vi "--Autonomous Independent.vi"() -> ()   [LabVIEW 2012]
doc: "This VI is called when autonomous begins, and will automatically be terminated when autonomous ends. You can carry out timed or sensor driven robot movement independently without needing to return to the caller."
uses:
  <vilib>/Rock Robotics/WPI/Relay/WPI_RelayValue.ctl
  <vilib>/Rock Robotics/WPI/Solenoid/WPI_SolenoidValue.ctl
  Robot Global Data.vi
  <vilib>/Rock Robotics/WPI/RobotDrive/WPI_RobotDriveGetSetRefNum.vi
  <vilib>/Rock Robotics/WPI/Solenoid/WPI_SolenoidSetEnum.vi
  <vilib>/Rock Robotics/WPI/Joystick/WPI_JoystickGetSetRefNum.vi
  <vilib>/addons/control/pid/NI_PID_pid.lvlib
  <vilib>/addons/control/pid/pid.llb/PID (DBL).vi
panel:
  in  "Auton Launch Reduction":dbl
  in  "Quicklaunch State":T1(ring)
  in  "Fast-Slow Variable":dbl
  out "Launch Wait tick":dbl
  out "Time Between tick":dbl
  in  "Time Between Launches":dbl=2000.0
  in  "Charge Up Time":dbl=4000.0
  out "Charge Up tick":dbl
  in  "Launch Wait Time":dbl=500.0
  in  "Turn wait time fr":dbl=250.0
  in  "Drive wait time fr":dbl=400.0
  in  "Turn wait time fl":dbl=250.0
  in  "Drive wait time fl":dbl=400.0
  in  "Drive wait time cl":dbl=400.0
  in  "Turn wait time cr":dbl=250.0
  in  "Drive wait time cr":dbl=400.0
  in  "Time between launches":dbl=1000.0
  in  "Launcher Charge time":dbl=5000.0
  in  "Drive PID gains":T2={"proportional gain (Kc)"=1.0, "integral time (Ti, min)"=0.01, "derivative time (Td, min)"=0.0} {"derivative time (Td, min)" format="%.3f"; "integral time (Ti, min)" format="%.3f"; "proportional gain (Kc)" format="%.3f"}
  in  "Turn wait time cl":dbl=250.0
  out "Field Position":enum16{"Corner", "Middle"}(ring)
  in  "Turn PID gains":T2={"proportional gain (Kc)"=1.0, "integral time (Ti, min)"=0.01, "derivative time (Td, min)"=0.0} {"derivative time (Td, min)" format="%.3f"; "integral time (Ti, min)" format="%.3f"; "proportional gain (Kc)" format="%.3f"}
  in  "Sweet Spot":dbl
  out "tick":dbl
  in  "-Fast-Slow Variable":dbl=2.0
  out "Numeric 0":dbl
  out "Current Movement, for debugging":T3 {"Y Joystick Value" scale=1.0..-1.0; "X Joystick Value" scale=-1.0..1.0}
  in  "Array of robot movements":T4(array[cluster]) {"Y Joystick Value" scale=1.0..-1.0; "X Joystick Value" scale=-1.0..1.0}
  # "Be sure to right-click and choose Data Operations>>Make Current Value default if you want to save the array values with the VI"
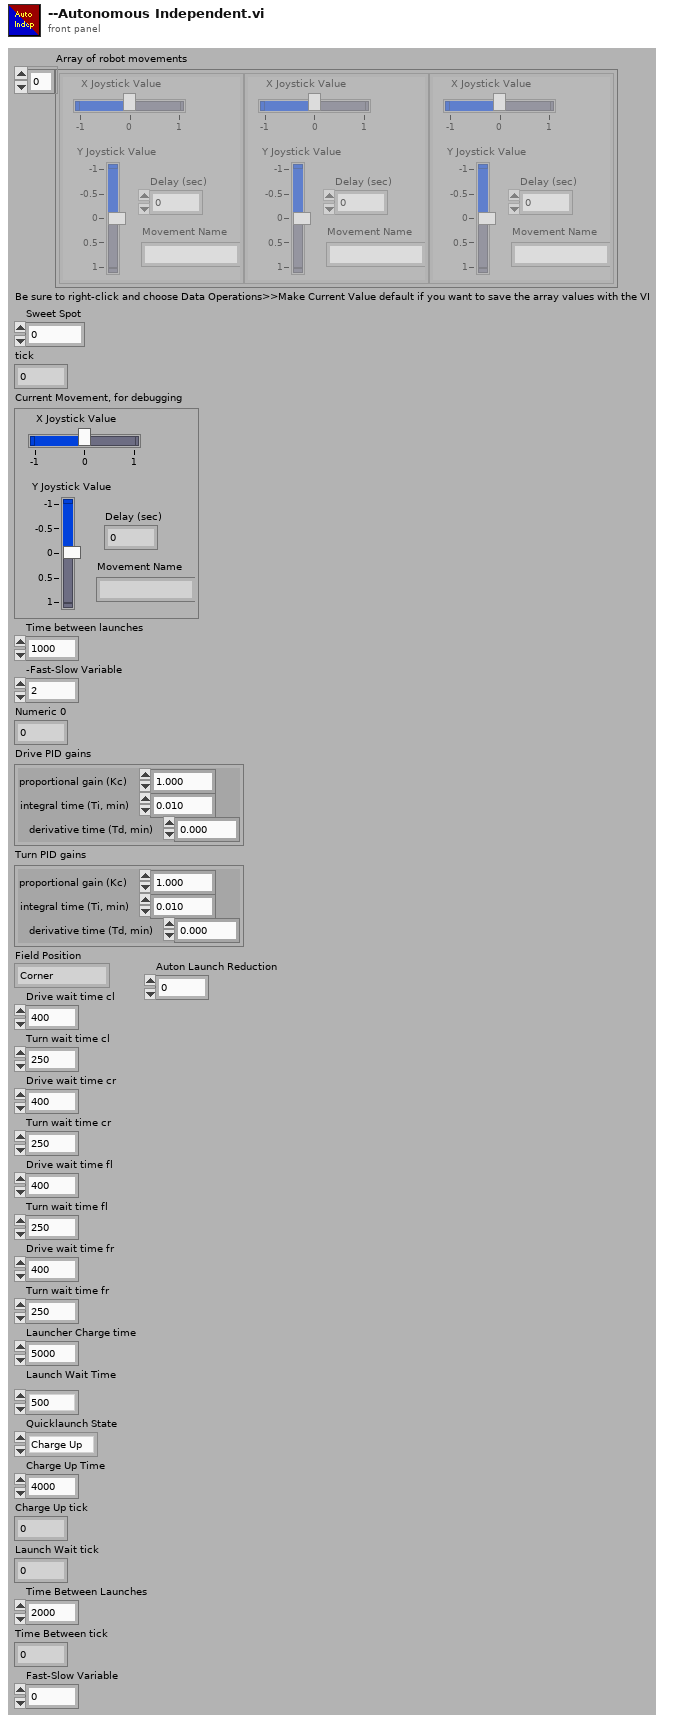
[diagram p1: front panel]
types:
  T1 = enum16{"Charge Up ", "Fire 1", "wait1", "Fire 2", "wait2", "Fire 3", "wait3", "Fire 4"}
  T2 = cluster{"proportional gain (Kc)":dbl, "integral time (Ti, min)":dbl, "derivative time (Td, min)":dbl}
  T3 = cluster{"X Joystick Value":dbl, "Y Joystick Value":dbl, "Delay (sec)":dbl, "Movement Name":string}
  T4 = cluster{"X Joystick Value":dbl, "Y Joystick Value":dbl, "Delay (sec)":dbl, "Movement Name":string}[]
  T5 = typedef "WPI_JoystickDevRef.ctl" = cluster{"Device":T6}
  T6 = typedef "WPI_JoystickDeviceEnum.ctl" = enum16{"USB 1", "USB 2", "USB 3", "USB 4", "Kinect 1", "Kinect 2"}
  T7 = cluster{"axis 1 (x)":dbl, "axis 2 (y)":dbl, "axis 3 (throttle)":dbl, "axis 4":dbl, "axis 5":dbl, "axis 6":dbl}
  T8 = typedef "WPI_SolenoidValue.ctl" = enum16{"Off", "On", "Forward", "Reverse"}
  T9 = typedef "WPI_RobotDriveDevRef.ctl" = cluster{"DevStatus":errorcluster, "Motors[]":T10[], "Square Inputs":bool, "Max Output":dbl, "Isochronous":bool}
  T10 = typedef "WPI_MotorControlDeviceRef.ctl" = cluster{"DeviceStatus":errorcluster, "Type":enum16{"PWM", "CAN"}, "PWM":cluster{"Digital Module":T11, "PWM Channel":T12, "DeadBand":T13}, "CAN":cluster{"Device Number":u8, "Control Mode":T14, "Semaphore":T15, "Max Vout":dbl}, "Invert":bool, "TransformRef":T16, "InvTransformRef":T16}
  T11 = typedef "FPGA_TypedefDigitalModule.ctl" = enum16{"Digital Module 1", "Digital Module 2"}
  T12 = typedef "FPGA_DIOPWMChannel.ctl" = enum8{"PWM 1", "PWM 2", "PWM 3", "PWM 4", "PWM 5", "PWM 6", "PWM 7", "PWM 8", "PWM 9", "PWM 10", "Invalid"}
  T13 = typedef "WPI_PWMDeadband.ctl" = cluster{"Name":string, "maxPositivePwm":i32, "minPositivePwm":i32, "centerPwm":i32, "maxNegativePwm":i32, "minNegativePwm":i32, "angularRange":u16}
  T14 = typedef "WPI_CANJaguar_ControlMode.ctl" = enum8{"Percent VBus", "Current", "Speed", "Position", "Voltage"}
  T15 = typedef "Semaphore RefNum" = refnum<k1>
  T16 = typedef "WPI_PWMTransform_ConPane.ctl" = refnum<vi>
  T17 = cluster{"Center Position":cluster{"X":dbl, "Y":dbl}, "Distance (ft)":dbl, "Center":bool}[]
  T18 = cluster{"Target Info[0]":cluster{"Center Position":cluster{"X":dbl, "Y":dbl}, "Distance (ft)":dbl, "Center":bool}, "Target Info[1]":cluster{"Center Position":cluster{"X":dbl, "Y":dbl}, "Distance (ft)":dbl, "Center":bool}, "Target Info[2]":cluster{"Center Position":cluster{"X":dbl, "Y":dbl}, "Distance (ft)":dbl, "Center":bool}, "Target Info[3]":cluster{"Center Position":cluster{"X":dbl, "Y":dbl}, "Distance (ft)":dbl, "Center":bool}, "Target Info[4]":cluster{"Center Position":cluster{"X":dbl, "Y":dbl}, "Distance (ft)":dbl, "Center":bool}, "Target Info[5]":cluster{"Center Position":cluster{"X":dbl, "Y":dbl}, "Distance (ft)":dbl, "Center":bool}, "Target Info[6]":cluster{"Center Position":cluster{"X":dbl, "Y":dbl}, "Distance (ft)":dbl, "Center":bool}, "Target Info[7]":cluster{"Center Position":cluster{"X":dbl, "Y":dbl}, "Distance (ft)":dbl, "Center":bool}, "Target Info[8]":cluster{"Center Position":cluster{"X":dbl, "Y":dbl}, "Distance (ft)":dbl, "Center":bool}}
  T19 = cluster{"Center Position":cluster{"X":dbl, "Y":dbl}, "Distance (ft)":dbl, "Center":bool}
  T20 = typedef "WPI_SolenoidDevRef.ctl" = cluster{"DevStatus":errorcluster, "Solenoid Module":T21, "Forward Solenoid Channel":T22, "Reverse Solenoid Channel":T22}
  T21 = typedef "FPGA_TypedefSolenoidModule.ctl" = enum16{"Solenoid Module 1", "Solenoid Module 2"}
  T22 = typedef "WPI_SolenoidChannel.ctl" = enum8{"Solenoid 1", "Solenoid 2", "Solenoid 3", "Solenoid 4", "Solenoid 5", "Solenoid 6", "Solenoid 7", "Solenoid 8", "Invalid"}
  T23 = typedef "WPI_RelayValue.ctl" = enum16{"Off", "On", "Forward", "Reverse"}
  T24 = typedef "WPI_RelayDevRef.ctl" = cluster{"DevStatus":errorcluster, "Relay Channel":T25, "Digital Module":T11, "Relay Direction":T26}
  T25 = typedef "FPGA_DIORelayChannel.ctl" = enum8{"Relay 1", "Relay 2", "Relay 3", "Relay 4", "Relay 5", "Relay 6", "Relay 7", "Relay 8", "Invalid"}
  T26 = typedef "WPI_RelayDirection.ctl" = enum16{"Both directions", "Forward only", "Reverse only"}
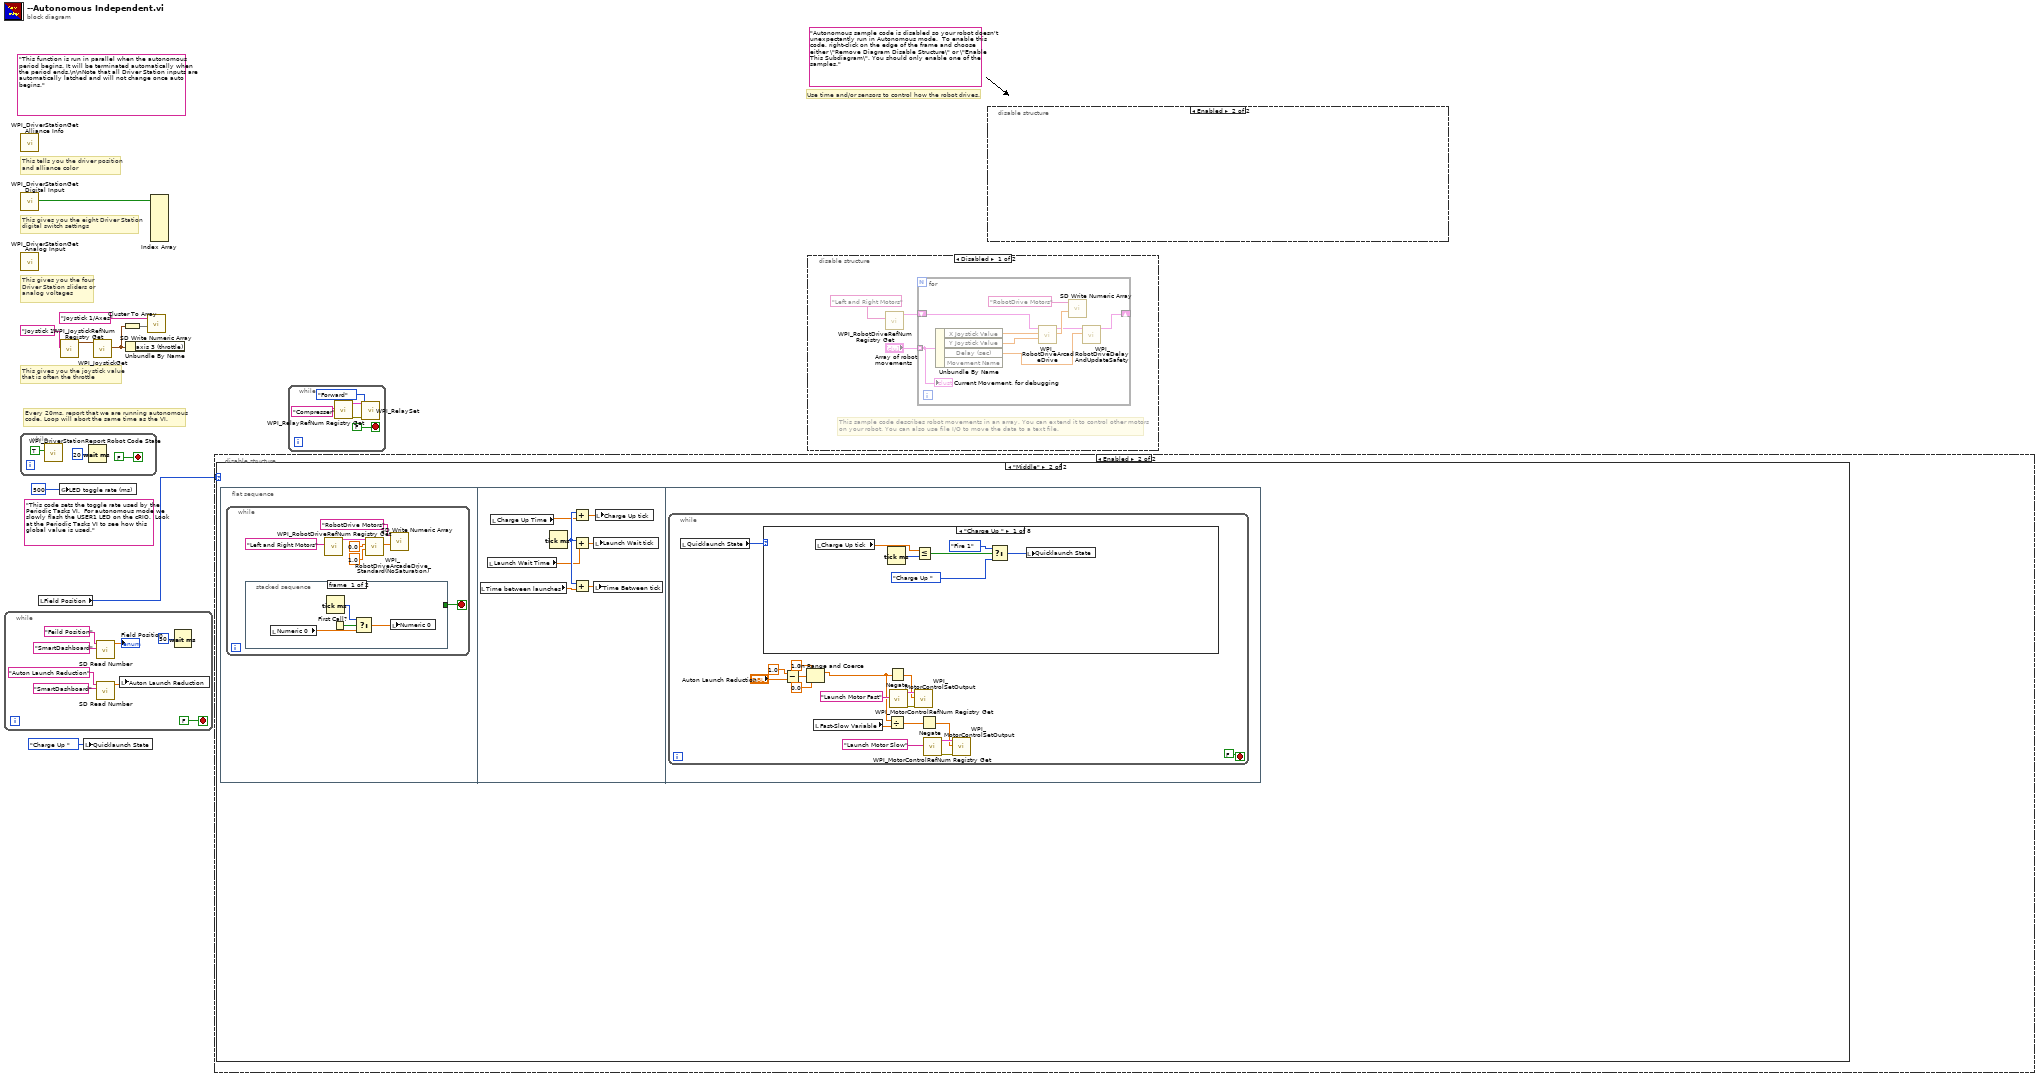
[diagram p0: block diagram]
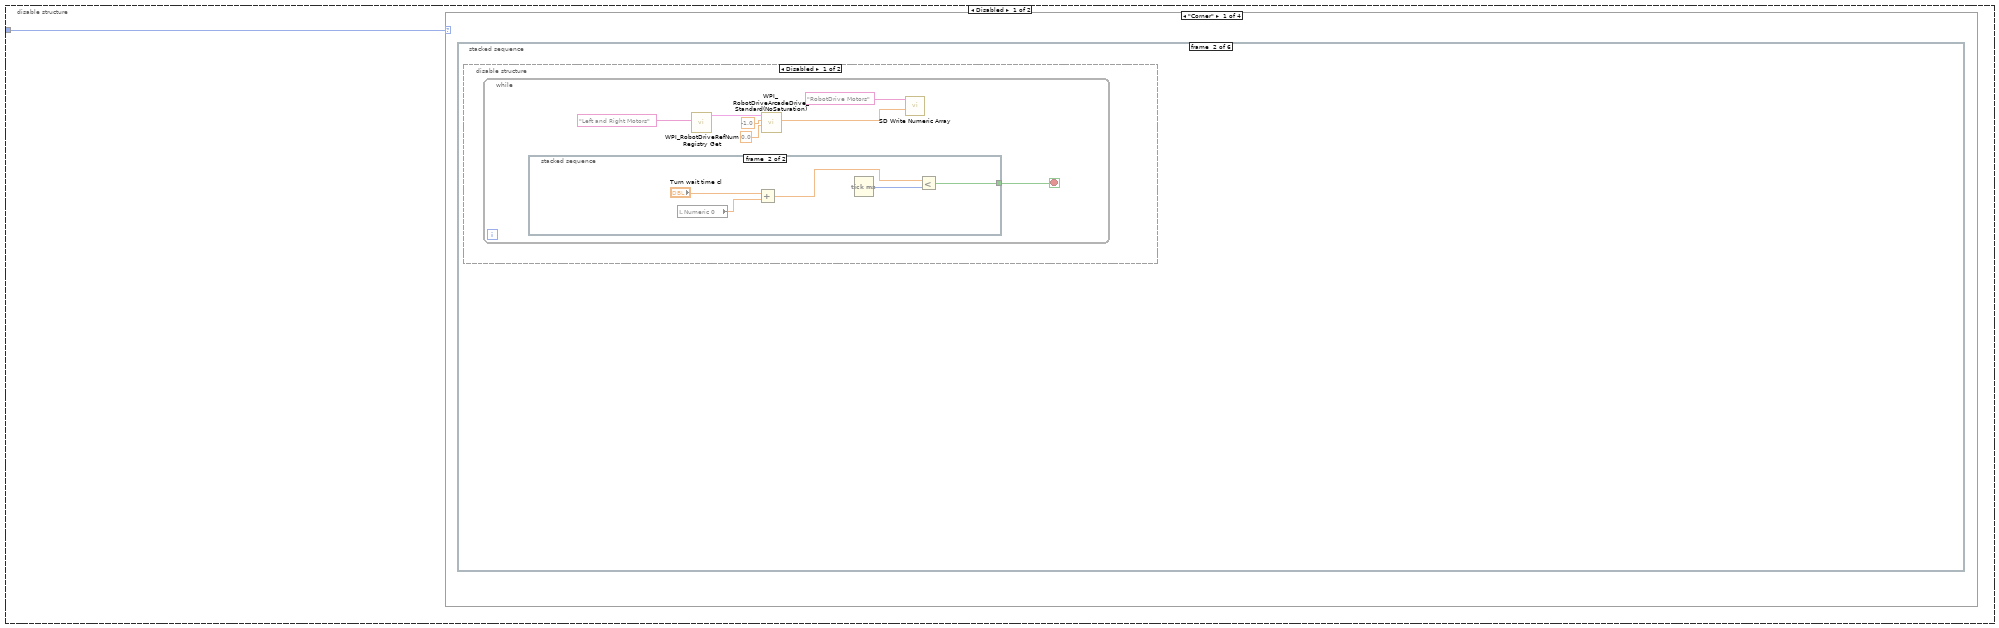
[diagram p2: hidden frame]
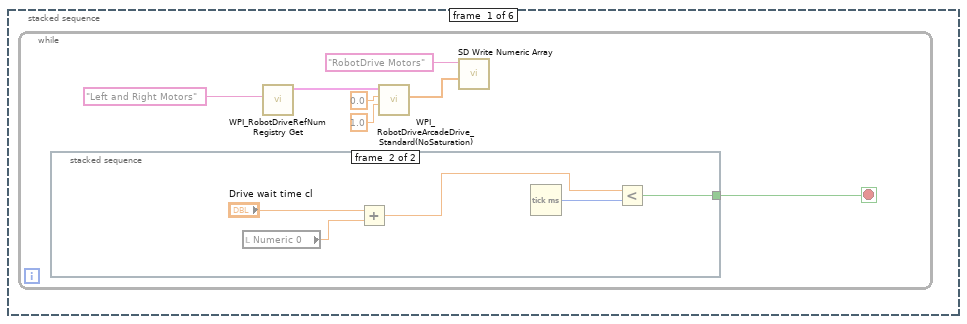
[diagram p3: hidden frame]
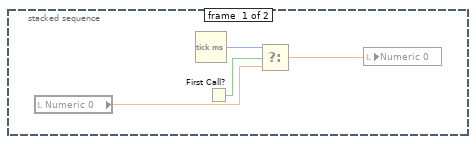
[diagram p4: hidden frame]
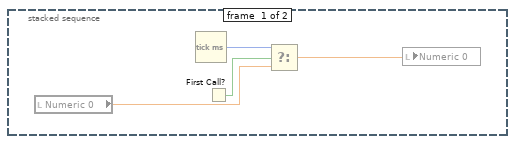
[diagram p5: hidden frame]
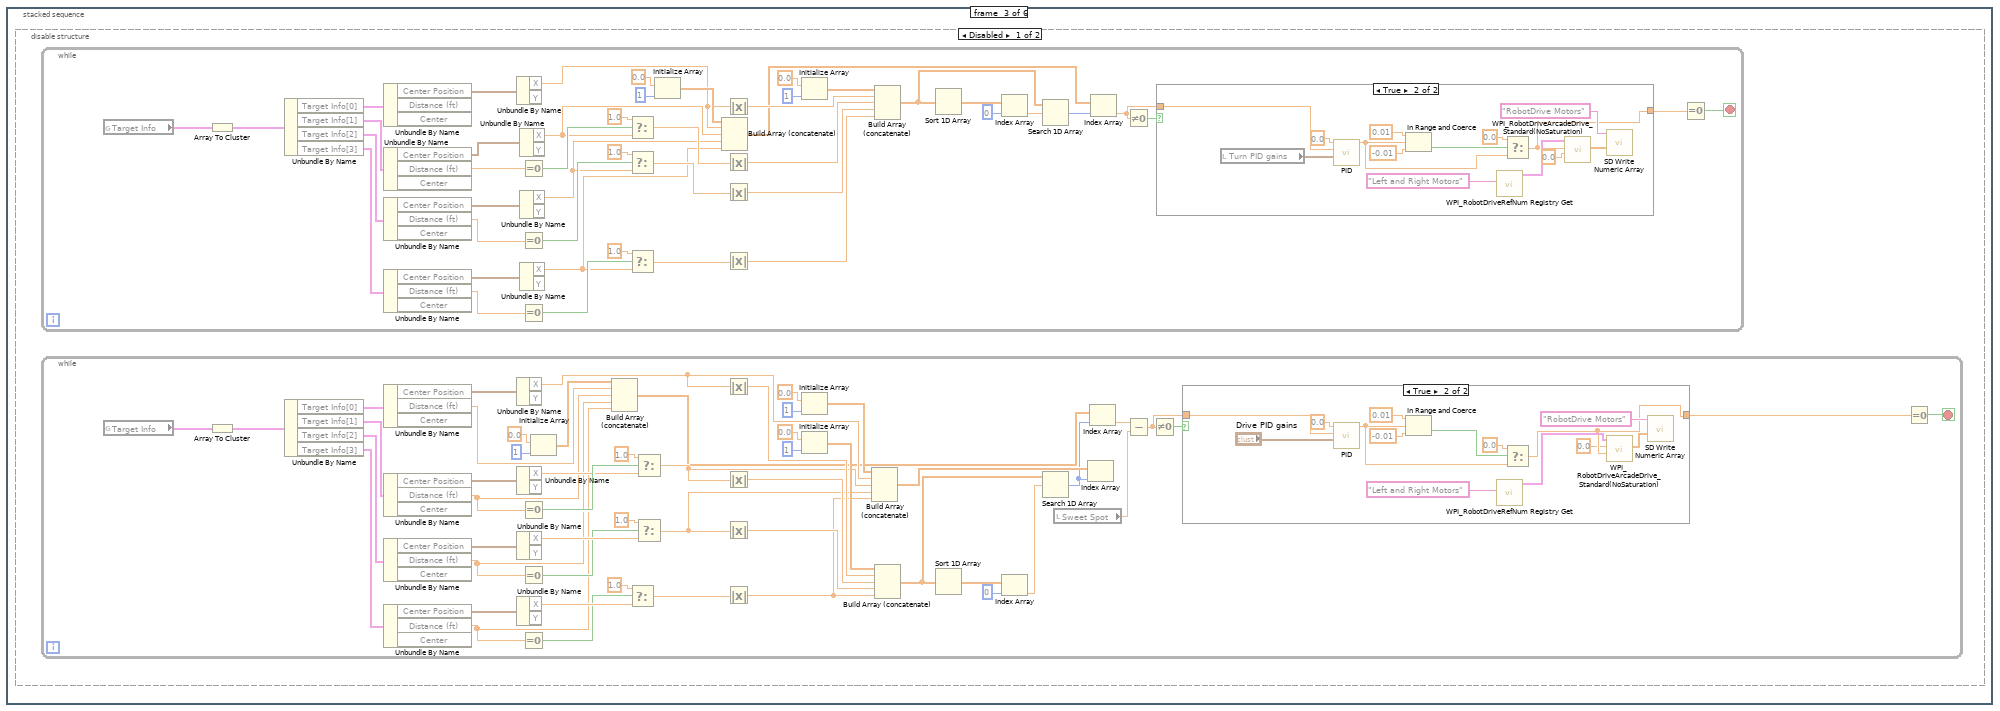
[diagram p7: hidden frame]
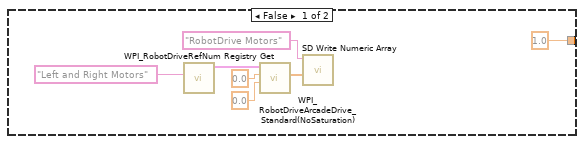
[diagram p8: hidden frame]
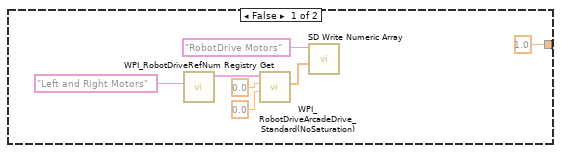
[diagram p9: hidden frame]
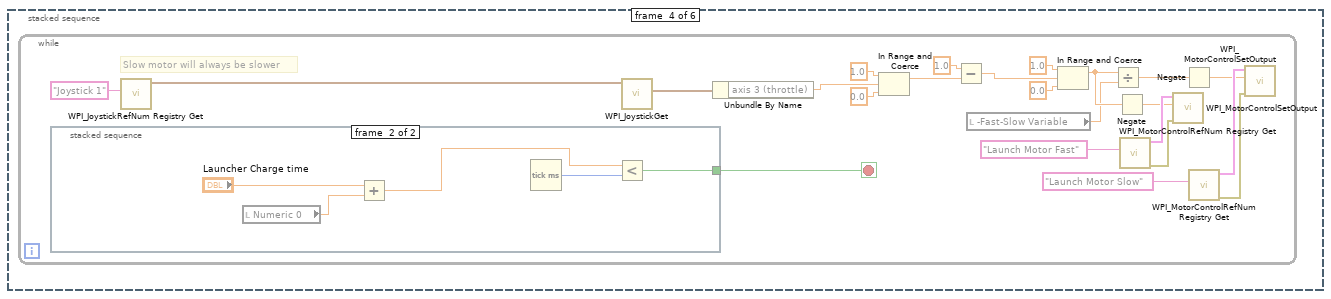
[diagram p11: hidden frame]
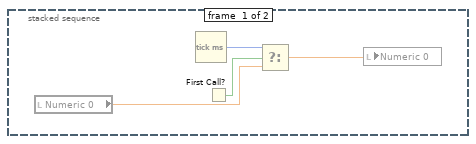
[diagram p12: hidden frame]
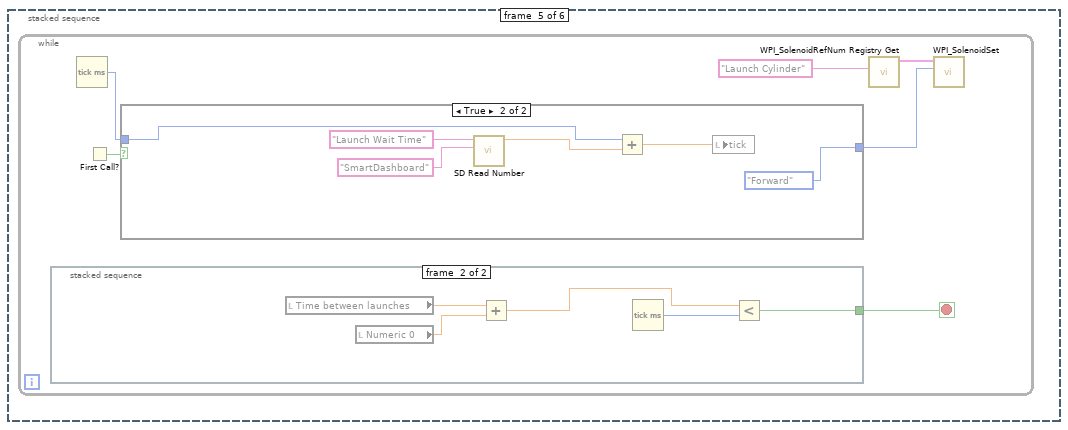
[diagram p13: hidden frame]
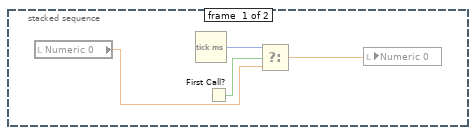
[diagram p14: hidden frame]
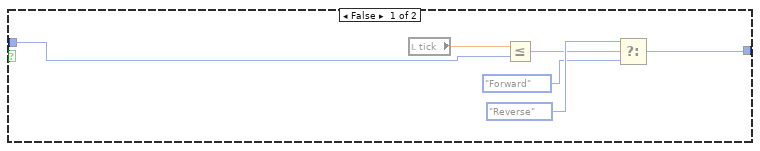
[diagram p15: hidden frame]
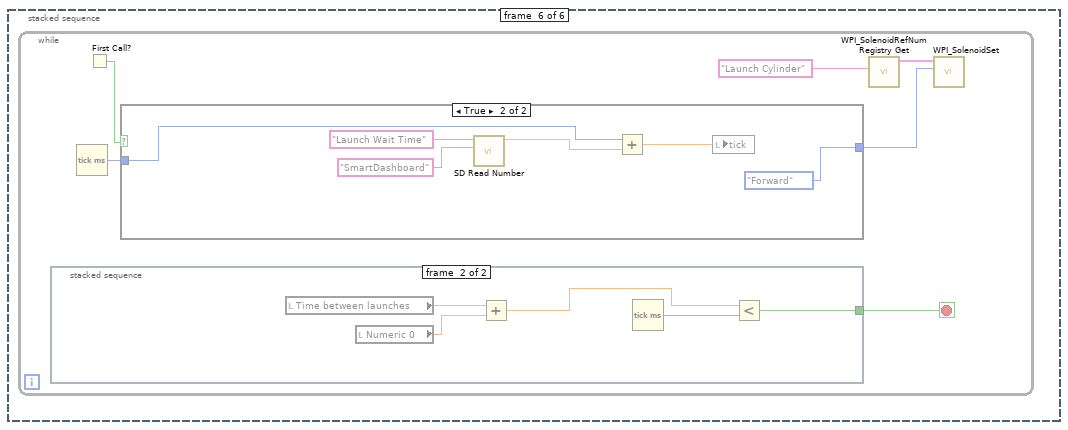
[diagram p16: hidden frame]
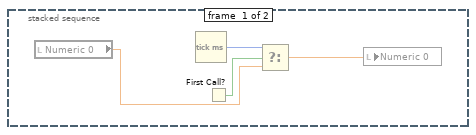
[diagram p17: hidden frame]
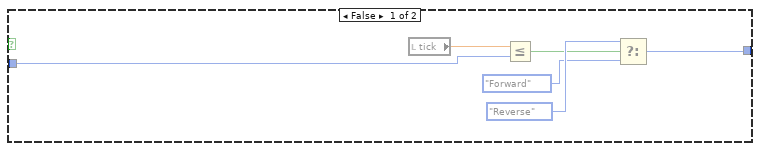
[diagram p18: hidden frame]
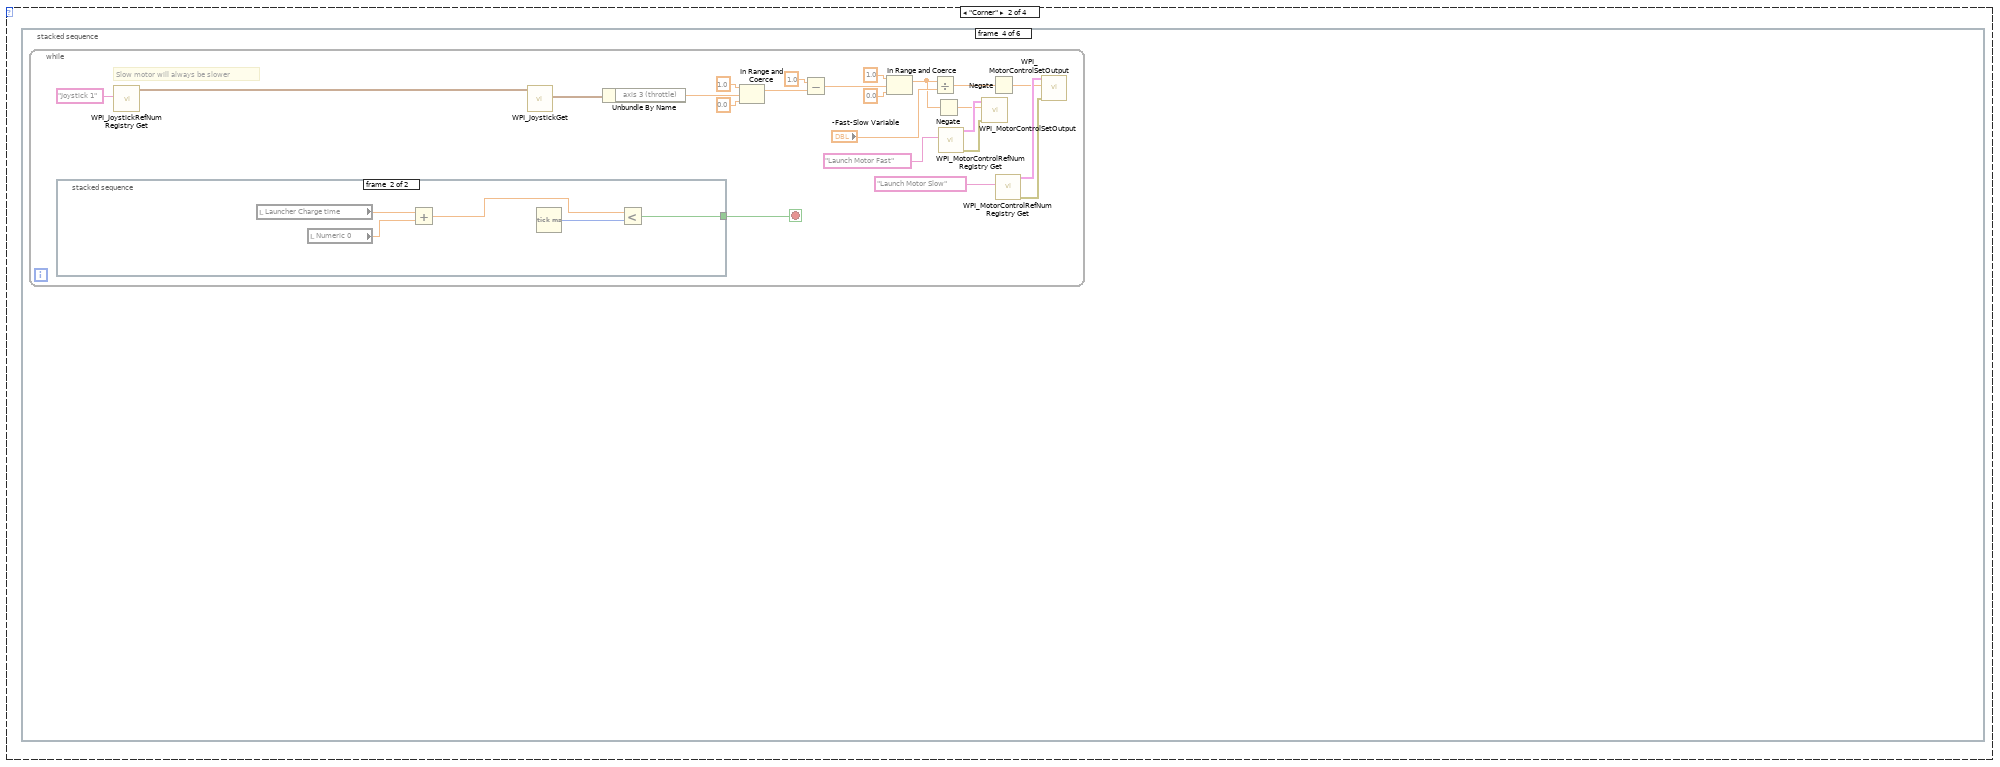
[diagram p19: hidden frame]
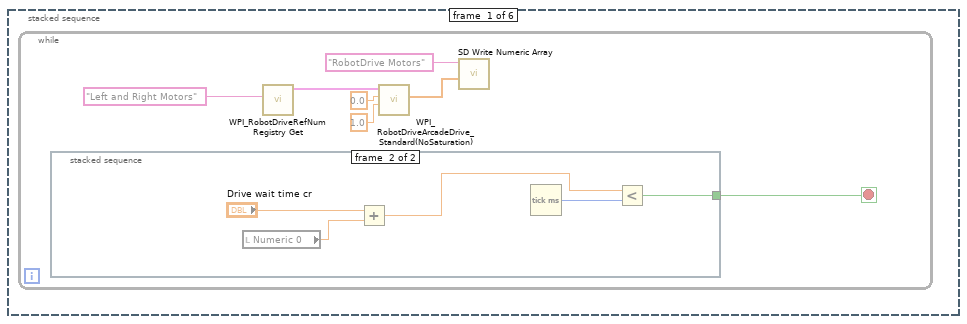
[diagram p20: hidden frame]
diagram:
  (unwired) "This code sets the toggle rate used by the Periodic Tasks VI.  For autonomous mode we slowly flash the USER1 LED on the cRIO.  Look at the Periodic Tasks VI to see how this global value is used."
  (unwired) "Autonomous sample code is disabled so your robot doesn't unexpectantly run in Autonomous mode.  To enable this code, right-click on the edge of the frame and choose either \"Remove Diagram Disable Structure\" or \"Enable This Subdiagram\". You should only enable one of the samples."
  (unwired) "This function is run in parallel when the autonomous period begins. It will be terminated automatically when the period ends.\n\nNote that all Driver Station inputs are automatically latched and will not change once auto begins."
  # "Every 20ms, report that we are running autonomous\ncode. Loop will abort the same time as the VI."
  # "This gives you the joystick value\nthat is often the throttle"
  # "Use time and/or sensors to control how the robot drives."
  # "This tells you the driver position\nand alliance color"
  # "This gives you the eight Driver Station\ndigital switch settings"
  # "This gives you the four\nDriver Station sliders or\nanalog voltages"
  n1 = while {
    stop <- FALSE stop-if-true
    n2 = call <vilib>:"SD Read Number.vi"("Table Prefix"="SmartDashboard", "Name"="Auton Launch Reduction") -> ("Numeric"=w12:dbl)  [unwired: 7 in, 2 out]
    n3 = call <vilib>:"SD Read Number.vi"("Table Prefix"="SmartDashboard", "Name"="Feild Position") -> ("Numeric"=→"Field Position":dbl)  [unwired: 7 in, 2 out]
    n4 = local write "Auton Launch Reduction"(w12) -> ()
    n5 = Wait (ms)(milliseconds to wait=u32 50) -> ()  [unwired: 1 out]
  }
  n6 = while {
    stop <- FALSE stop-if-true
    n7 = call <vilib>:"WPI_DriverStationReport Robot Code State.vi"("Autonomous"=TRUE) -> ()  [unwired: 10 in, 1 out]
    n8 = Wait (ms)(milliseconds to wait=u32 20) -> ()  [unwired: 1 out]
  }
  n9 = call <vilib>:"WPI_DriverStationGet Alliance Info.vi"() -> ()  [unwired: 12 out]
  n10 = call <vilib>:"WPI_DriverStationGet Digital Input.vi"() -> ("Driver Station Digital Input (1-8)"=w9:bool[])  [unwired: 11 out]
  n11 = call <vilib>:"WPI_DriverStationGet Analog Input.vi"() -> ()  [unwired: 12 out]
  n12 = local read "Field Position"() -> (w2:enum16{"Corner", "Middle"})
  n13 = global write "Robot Global Data.vi" "LED toggle rate (ms)"(u32 500 ("LED ms toggle rate")) -> ()
  n14 = call <vilib>:"WPI_JoystickRefNum Registry Get.vi"("refnum name"="Joystick 1") -> ("JoystickDevRef"=w7:T5)  [unwired: 1 in, 9 out]
  n15 = local write "Quicklaunch State"(T1."Charge Up " ("Quicklaunch State")) -> ()
  n16 = call <vilib>:"WPI_JoystickGet.vi"("JoystickDevRef"=w7) -> ("Axes"=w4:T7)  [unwired: 1 in, 5 out]
  n17 = Cluster To Array(cluster=w4) -> (array=w5:dbl[])
  n18 = Unbundle By Name(w4) -> ()  [unwired: 1 out]
  n19 = call <vilib>:"SD Write Numeric Array.vi"("Numeric Array"=w5, "Name"="Joystick 1/Axes") -> ()  [unwired: 8 in, 2 out]
  n20 = Index Array(array=w9) -> ()  [unwired: 8 in, 8 out]
  n21 = disable-structure shown="Enabled" {
    disable-tunnel: w2 -> [w21 w1108]
    frame Disabled {
      n22 = case shown="\"Far Right\"" w21 {
        frame "Corner" {
          n23 = stacked-sequence {
            frame #0 {
              n24 = while {
                stop <- w22 stop-if-true
                n25 = stacked-sequence {
                  tunnel: [_ w34] -> w22
                  frame #0 {
                    n26 = local read "Numeric 0"() -> (w30:dbl)
                    n27 = Tick Count (ms)() -> (millisecond timer value=w31:u32)
                    n28 = First Call?() -> (First Call?: T/F=w32:bool)
                    n29 = Select(t=w31, s=w32, f=w30) -> (s? t:f=w29:dbl)
                    n30 = local write "Numeric 0"(w29) -> ()
                  }
                  frame #1 {
                    n31 = local read "Numeric 0"() -> (w37:dbl)
                    n32 = Add(x="Drive wait time cl", y=w37) -> (x+y=w36:dbl)
                    n33 = Tick Count (ms)() -> (millisecond timer value=w35:u32)
                    n34 = Less?(x=w36, y=w35) -> (x < y?=w34:bool)
                  }
                }
                n35 = call <vilib>:"WPI_RobotDriveRefNum Registry Get.vi"("refnum name"="Left and Right Motors") -> ("RobotDriveDevRef"=w27:T9)  [unwired: 1 in, 9 out]
                n36 = call <vilib>:"WPI_RobotDriveArcadeDrive_Standard(NoSaturation).vi"("Y axis value"=1.0 ("X axis value"), "X axis value"=0.0, "RobotDriveDevRef"=w27) -> ("Motor Values"=w25:dbl[])  [unwired: 1 in, 7 out]
                n37 = call <vilib>:"SD Write Numeric Array.vi"("Numeric Array"=w25, "Name"="RobotDrive Motors") -> ()  [unwired: 8 in, 2 out]
              }
            }
            frame #1 {
              n38 = disable-structure shown="Disabled" {
                frame Disabled {
                  n39 = while {
                    stop <- w38 stop-if-true
                    n40 = stacked-sequence {
                      tunnel: [_ w50] -> w38
                      frame #0 {
                        n41 = local read "Numeric 0"() -> (w46:dbl)
                        n42 = Tick Count (ms)() -> (millisecond timer value=w47:u32)
                        n43 = First Call?() -> (First Call?: T/F=w48:bool)
                        n44 = Select(t=w47, s=w48, f=w46) -> (s? t:f=w45:dbl)
                        n45 = local write "Numeric 0"(w45) -> ()
                      }
                      frame #1 {
                        n46 = local read "Numeric 0"() -> (w53:dbl)
                        n47 = Add(x="Turn wait time cl", y=w53) -> (x+y=w52:dbl)
                        n48 = Tick Count (ms)() -> (millisecond timer value=w51:u32)
                        n49 = Less?(x=w52, y=w51) -> (x < y?=w50:bool)
                      }
                    }
                    n50 = call <vilib>:"WPI_RobotDriveRefNum Registry Get.vi"("refnum name"="Left and Right Motors") -> ("RobotDriveDevRef"=w40:T9)  [unwired: 1 in, 9 out]
                    n51 = call <vilib>:"WPI_RobotDriveArcadeDrive_Standard(NoSaturation).vi"("Y axis value"=0.0 ("X axis value"), "X axis value"=-1.0, "RobotDriveDevRef"=w40) -> ("Motor Values"=w42:dbl[])  [unwired: 1 in, 7 out]
                    n52 = call <vilib>:"SD Write Numeric Array.vi"("Numeric Array"=w42, "Name"="RobotDrive Motors") -> ()  [unwired: 8 in, 2 out]
                  }
                }
                frame Enabled {
                }
              }
            }
            frame #2 {
              n53 = disable-structure shown="Disabled" {
                frame Disabled {
                  n54 = while {
                    stop <- w81 stop-if-true
                    n55 = global read "Robot Global Data.vi" "Target Info"() -> (w99:T17)
                    n56 = Array To Cluster(array=w99) -> (cluster=w98:T18)
                    n57 = Unbundle By Name(w98) -> ("Target Info[0]"=w97:T19, "Target Info[1]"=w92:T19, "Target Info[2]"=w91:T19, "Target Info[3]"=w90:T19)
                    n58 = Unbundle By Name(w97) -> ("Center Position"=w96:cluster{"X":dbl, "Y":dbl})  [unwired: 2 out]
                    n59 = Unbundle By Name(w92) -> ("Center Position"=w95:cluster{"X":dbl, "Y":dbl}, "Distance (ft)"=w58:dbl)  [unwired: 1 out]
                    n60 = Unbundle By Name(w91) -> ("Center Position"=w94:cluster{"X":dbl, "Y":dbl}, "Distance (ft)"=w60:dbl)  [unwired: 1 out]
                    n61 = Unbundle By Name(w90) -> ("Center Position"=w93:cluster{"X":dbl, "Y":dbl}, "Distance (ft)"=w62:dbl)  [unwired: 1 out]
                    n62 = Unbundle By Name(w96) -> ("X"=w56:dbl)  [unwired: 1 out]
                    n63 = Unbundle By Name(w95) -> ("X"=w57:dbl)  [unwired: 1 out]
                    n64 = Unbundle By Name(w94) -> ("X"=w59:dbl)  [unwired: 1 out]
                    n65 = Unbundle By Name(w93) -> ("X"=w61:dbl)  [unwired: 1 out]
                    n66 = Equal To 0?(x=w58) -> (x = 0?=w89:bool)
                    n67 = Equal To 0?(x=w60) -> (x = 0?=w88:bool)
                    n68 = Equal To 0?(x=w62) -> (x = 0?=w87:bool)
                    n69 = Select(t=1.0, s=w89, f=w57) -> (s? t:f=w70:dbl)
                    n70 = Select(t=1.0, s=w88, f=w59) -> (s? t:f=w69:dbl)
                    n71 = Select(t=1.0, s=w87, f=w61) -> (s? t:f=w83:dbl)
                    n72 = Initialize Array(0.0 ("element"), 1 ("dimension size")) -> (w65:dbl[])
                    n73 = Build Array (concatenate)(w65, w56, w57, w59, w61) -> (w64:dbl[])
                    n74 = Absolute Value(x=w56) -> (abs(x)=w77:dbl)
                    n75 = Absolute Value(x=w70) -> (abs(x)=w76:dbl)
                    n76 = Absolute Value(x=w69) -> (abs(x)=w75:dbl)
                    n77 = Absolute Value(x=w83) -> (abs(x)=w68:dbl)
                    n78 = Initialize Array(0.0 ("element"), 1 ("dimension size")) -> (w78:dbl[])
                    n79 = Build Array (concatenate)(w78, w77, w76, w75, w68) -> (w71:dbl[])
                    n80 = Sort 1D Array(array=w71) -> (sorted array=w74:dbl[])
                    n81 = Index Array(array=w74, index=0) -> (element=w72:dbl)
                    n82 = Search 1D Array(1D array=w71, element=w72) -> (index of element=w63:i32)  [unwired: 1 in]
                    n83 = Index Array(array=w64, index=w63) -> (element=w54:dbl)
                    n84 = Not Equal To 0?(x=w54) -> (x != 0?=w55:bool)
                    n85 = case shown="True" w55 {
                      tunnel: [1.0 ("output") w109] -> w82
                      tunnel: w54 -> [_ w108]
                      frame False {
                        n86 = call <vilib>:"WPI_RobotDriveRefNum Registry Get.vi"("refnum name"="Left and Right Motors") -> ("RobotDriveDevRef"=w105:T9)  [unwired: 1 in, 9 out]
                        n87 = call <vilib>:"WPI_RobotDriveArcadeDrive_Standard(NoSaturation).vi"("Y axis value"=0.0, "X axis value"=0.0, "RobotDriveDevRef"=w105) -> ("Motor Values"=w103:dbl[])  [unwired: 1 in, 7 out]
                        n88 = call <vilib>:"SD Write Numeric Array.vi"("Numeric Array"=w103, "Name"="RobotDrive Motors") -> ()  [unwired: 8 in, 2 out]
                      }
                      frame True {
                        n89 = local read "Turn PID gains"() -> (w107:T2)
                        n90 = call-poly <vilib>:"PID.vi"("PID gains"=w107, "process variable"=w108, "setpoint"=0.0 ("process variable")) -> ("output"=w110:dbl)  [unwired: 7 in, 1 out]
                        n91 = In Range and Coerce(upper limit=0.01, x=w110, lower limit=-0.01) -> (In Range?=w112:bool)  [unwired: 1 out]
                        n92 = call <vilib>:"WPI_RobotDriveRefNum Registry Get.vi"("refnum name"="Left and Right Motors") -> ("RobotDriveDevRef"=w118:T9)  [unwired: 1 in, 9 out]
                        n93 = Select(t=0.0, s=w112, f=w110) -> (s? t:f=w109:dbl)
                        n94 = call <vilib>:"WPI_RobotDriveArcadeDrive_Standard(NoSaturation).vi"("Y axis value"=0.0, "X axis value"=w109, "RobotDriveDevRef"=w118) -> ("Motor Values"=w117:dbl[])  [unwired: 1 in, 7 out]
                        n95 = call <vilib>:"SD Write Numeric Array.vi"("Numeric Array"=w117, "Name"="RobotDrive Motors") -> ()  [unwired: 8 in, 2 out]
                      }
                    }
                    n96 = Equal To 0?(x=w82) -> (x = 0?=w81:bool)
                  }
                  n97 = while {
                    stop <- w152 stop-if-true
                    n98 = global read "Robot Global Data.vi" "Target Info"() -> (w173:T17)
                    n99 = Array To Cluster(array=w173) -> (cluster=w172:T18)
                    n100 = Unbundle By Name(w172) -> ("Target Info[0]"=w171:T19, "Target Info[1]"=w166:T19, "Target Info[2]"=w165:T19, "Target Info[3]"=w164:T19)
                    n101 = Unbundle By Name(w171) -> ("Center Position"=w170:cluster{"X":dbl, "Y":dbl}, "Distance (ft)"=w130:dbl)  [unwired: 1 out]
                    n102 = Unbundle By Name(w166) -> ("Center Position"=w169:cluster{"X":dbl, "Y":dbl}, "Distance (ft)"=w129:dbl)  [unwired: 1 out]
                    n103 = Unbundle By Name(w165) -> ("Center Position"=w168:cluster{"X":dbl, "Y":dbl}, "Distance (ft)"=w128:dbl)  [unwired: 1 out]
                    n104 = Unbundle By Name(w164) -> ("Center Position"=w167:cluster{"X":dbl, "Y":dbl}, "Distance (ft)"=w127:dbl)  [unwired: 1 out]
                    n105 = Unbundle By Name(w170) -> ("X"=w138:dbl)  [unwired: 1 out]
                    n106 = Unbundle By Name(w169) -> ("X"=w155:dbl)  [unwired: 1 out]
                    n107 = Unbundle By Name(w168) -> ("X"=w162:dbl)  [unwired: 1 out]
                    n108 = Unbundle By Name(w167) -> ("X"=w163:dbl)  [unwired: 1 out]
                    n109 = Equal To 0?(x=w129) -> (x = 0?=w161:bool)
                    n110 = Equal To 0?(x=w128) -> (x = 0?=w160:bool)
                    n111 = Equal To 0?(x=w127) -> (x = 0?=w159:bool)
                    n112 = Initialize Array(0.0 ("element"), 1 ("dimension size")) -> (w131:dbl[])
                    n113 = Build Array (concatenate)(w131, w130, w129, w128, w127) -> (w126:dbl[])
                    n114 = Select(t=1.0, s=w159, f=w163) -> (s? t:f=w154:dbl)
                    n115 = Select(t=1.0, s=w161, f=w155) -> (s? t:f=w137:dbl)
                    n116 = Select(t=1.0, s=w160, f=w162) -> (s? t:f=w136:dbl)
                    n117 = Absolute Value(x=w138) -> (abs(x)=w148:dbl)
                    n118 = Absolute Value(x=w137) -> (abs(x)=w147:dbl)
                    n119 = Absolute Value(x=w136) -> (abs(x)=w146:dbl)
                    n120 = Absolute Value(x=w154) -> (abs(x)=w135:dbl)
                    n121 = Initialize Array(0.0 ("element"), 1 ("dimension size")) -> (w139:dbl[])
                    n122 = Initialize Array(0.0 ("element"), 1 ("dimension size")) -> (w149:dbl[])
                    n123 = Build Array (concatenate)(w139, w138, w137, w136, w135) -> (w134:dbl[])
                    n124 = Build Array (concatenate)(w149, w148, w147, w146, w135) -> (w142:dbl[])
                    n125 = Sort 1D Array(array=w142) -> (sorted array=w145:dbl[])
                    n126 = Index Array(array=w145, index=0) -> (element=w143:dbl)
                    n127 = Search 1D Array(1D array=w142, element=w143) -> (index of element=w125:i32)  [unwired: 1 in]
                    n128 = local read "Sweet Spot"() -> (w121:dbl)
                    n129 = Index Array(array=w134, index=w125) -> ()  [unwired: 1 out]
                    n130 = Index Array(array=w126, index=w125) -> (element=w124:dbl)
                    n131 = Subtract(x=w124, y=w121) -> (x-y=w123:dbl)
                    n132 = Not Equal To 0?(x=w123) -> (x != 0?=w122:bool)
                    n133 = case shown="True" w122 {
                      tunnel: [1.0 ("output") w183] -> w153
                      tunnel: w123 -> [_ w184]
                      frame False {
                        n134 = call <vilib>:"WPI_RobotDriveRefNum Registry Get.vi"("refnum name"="Left and Right Motors") -> ("RobotDriveDevRef"=w179:T9)  [unwired: 1 in, 9 out]
                        n135 = call <vilib>:"WPI_RobotDriveArcadeDrive_Standard(NoSaturation).vi"("Y axis value"=0.0, "X axis value"=0.0, "RobotDriveDevRef"=w179) -> ("Motor Values"=w177:dbl[])  [unwired: 1 in, 7 out]
                        n136 = call <vilib>:"SD Write Numeric Array.vi"("Numeric Array"=w177, "Name"="RobotDrive Motors") -> ()  [unwired: 8 in, 2 out]
                      }
                      frame True {
                        n137 = call-poly <vilib>:"PID.vi"("PID gains"="Drive PID gains", "process variable"=w184, "setpoint"=0.0 ("process variable")) -> ("output"=w185:dbl)  [unwired: 7 in, 1 out]
                        n138 = In Range and Coerce(upper limit=0.01, x=w185, lower limit=-0.01) -> (In Range?=w187:bool)  [unwired: 1 out]
                        n139 = call <vilib>:"WPI_RobotDriveRefNum Registry Get.vi"("refnum name"="Left and Right Motors") -> ("RobotDriveDevRef"=w192:T9)  [unwired: 1 in, 9 out]
                        n140 = Select(t=0.0, s=w187, f=w185) -> (s? t:f=w183:dbl)
                        n141 = call <vilib>:"WPI_RobotDriveArcadeDrive_Standard(NoSaturation).vi"("Y axis value"=w183, "X axis value"=0.0, "RobotDriveDevRef"=w192) -> ("Motor Values"=w191:dbl[])  [unwired: 1 in, 7 out]
                        n142 = call <vilib>:"SD Write Numeric Array.vi"("Numeric Array"=w191, "Name"="RobotDrive Motors") -> ()  [unwired: 8 in, 2 out]
                      }
                    }
                    n143 = Equal To 0?(x=w153) -> (x = 0?=w152:bool)
                  }
                }
                frame Enabled {
                }
              }
            }
            frame #3 {
              n144 = while {
                stop <- w214 stop-if-true
                # "Slow motor will always be slower"
                n145 = stacked-sequence {
                  tunnel: [_ w223] -> w214
                  frame #0 {
                    n146 = local read "Numeric 0"() -> (w219:dbl)
                    n147 = Tick Count (ms)() -> (millisecond timer value=w220:u32)
                    n148 = First Call?() -> (First Call?: T/F=w221:bool)
                    n149 = Select(t=w220, s=w221, f=w219) -> (s? t:f=w218:dbl)
                    n150 = local write "Numeric 0"(w218) -> ()
                  }
                  frame #1 {
                    n151 = local read "Numeric 0"() -> (w226:dbl)
                    n152 = Add(x="Launcher Charge time", y=w226) -> (x+y=w225:dbl)
                    n153 = Tick Count (ms)() -> (millisecond timer value=w224:u32)
                    n154 = Less?(x=w225, y=w224) -> (x < y?=w223:bool)
                  }
                }
                n155 = call <vilib>:"WPI_JoystickRefNum Registry Get.vi"("refnum name"="Joystick 1") -> ("JoystickDevRef"=w216:T5)  [unwired: 1 in, 9 out]
                n156 = call <vilib>:"WPI_JoystickGet.vi"("JoystickDevRef"=w216) -> ("Axes"=w217:T7)  [unwired: 1 in, 5 out]
                n157 = Unbundle By Name(w217) -> ("axis 3 (throttle)"=w195:dbl)
                n158 = In Range and Coerce(upper limit=1.0, x=w195, lower limit=0.0) -> (coerced(x)=w200:dbl)  [unwired: 1 out]
                n159 = Subtract(x=1.0, y=w200) -> (x-y=w211:dbl)
                n160 = local read "-Fast-Slow Variable"() -> (w196:dbl)
                n161 = In Range and Coerce(upper limit=1.0, x=w211, lower limit=0.0) -> (coerced(x)=w197:dbl)  [unwired: 1 out]
                n162 = Divide(x=w197, y=w196) -> (x/y=w209:dbl)
                n163 = Negate(x=w197) -> (-x=w199:dbl)
                n164 = call <vilib>:"WPI_MotorControlRefNum Registry Get.vi"("refnum name"="Launch Motor Fast") -> ("error out"=w207:errorcluster, "MotorControlDevRef"=w206:T10)  [unwired: 9 in]
                n165 = call <vilib>:"WPI_MotorControlSetOutput.vi"("error in (no error)"=w207, "Output"=w199, "MotorControlDevRef"=w206) -> ()  [unwired: 6 in, 3 out]
                n166 = Negate(x=w209) -> (-x=w198:dbl)
                n167 = call <vilib>:"WPI_MotorControlRefNum Registry Get.vi"("refnum name"="Launch Motor Slow") -> ("error out"=w204:errorcluster, "MotorControlDevRef"=w205:T10)  [unwired: 9 in]
                n168 = call <vilib>:"WPI_MotorControlSetOutput.vi"("error in (no error)"=w204, "Output"=w198, "MotorControlDevRef"=w205) -> ()  [unwired: 6 in, 3 out]
              }
            }
            frame #4 {
              n169 = while {
                stop <- w227 stop-if-true
                n170 = stacked-sequence {
                  tunnel: [_ w238] -> w227
                  frame #0 {
                    n171 = local read "Numeric 0"() -> (w234:dbl)
                    n172 = Tick Count (ms)() -> (millisecond timer value=w235:u32)
                    n173 = First Call?() -> (First Call?: T/F=w236:bool)
                    n174 = Select(t=w235, s=w236, f=w234) -> (s? t:f=w233:dbl)
                    n175 = local write "Numeric 0"(w233) -> ()
                  }
                  frame #1 {
                    n176 = local read "Time between launches"() -> (w237:dbl)
                    n177 = local read "Numeric 0"() -> (w241:dbl)
                    n178 = Add(x=w237, y=w241) -> (x+y=w240:dbl)
                    n179 = Tick Count (ms)() -> (millisecond timer value=w239:u32)
                    n180 = Less?(x=w240, y=w239) -> (x < y?=w238:bool)
                  }
                }
                n181 = Tick Count (ms)() -> (millisecond timer value=w228:u32)
                n182 = First Call?() -> (First Call?: T/F=w232:bool)
                n183 = case shown="True" w232 {
                  tunnel: w228 -> [w246 w253]
                  tunnel: [w242 WPI_SolenoidValue."Forward" ("Value")] -> w231
                  frame False {
                    n184 = local read "tick"() -> (w247:dbl)
                    n185 = Less Or Equal?(x=w247, y=w246) -> (x <= y?=w243:bool)
                    n186 = Select(t=WPI_SolenoidValue."Reverse" ("Value"), s=w243, f=WPI_SolenoidValue."Forward" ("Value")) -> (s? t:f=w242:T8)
                  }
                  frame True {
                    n187 = call <vilib>:"SD Read Number.vi"("Table Prefix"="SmartDashboard", "Name"="Launch Wait Time") -> ("Numeric"=w248:dbl)  [unwired: 7 in, 2 out]
                    n188 = Add(x=w253, y=w248) -> (x+y=w251:dbl)
                    n189 = local write "tick"(w251) -> ()
                  }
                }
                n190 = call <vilib>:"WPI_SolenoidRefNum Registry Get.vi"("refnum name"="Launch Cylinder") -> ("SolenoidDevRef"=w230:T20)  [unwired: 9 in, 1 out]
                n191 = call-poly <vilib>:"WPI_SolenoidSet.vi"("Value"=w231, "SolenoidDevRef"=w230) -> ()  [unwired: 8 in, 2 out]
              }
            }
            frame #5 {
              n192 = while {
                stop <- w254 stop-if-true
                n193 = stacked-sequence {
                  tunnel: [_ w266] -> w254
                  frame #0 {
                    n194 = local read "Numeric 0"() -> (w261:dbl)
                    n195 = Tick Count (ms)() -> (millisecond timer value=w262:u32)
                    n196 = First Call?() -> (First Call?: T/F=w263:bool)
                    n197 = Select(t=w262, s=w263, f=w261) -> (s? t:f=w260:dbl)
                    n198 = local write "Numeric 0"(w260) -> ()
                  }
                  frame #1 {
                    n199 = local read "Time between launches"() -> (w264:dbl)
                    n200 = local read "Numeric 0"() -> (w265:dbl)
                    n201 = Add(x=w264, y=w265) -> (x+y=w268:dbl)
                    n202 = Tick Count (ms)() -> (millisecond timer value=w267:u32)
                    n203 = Less?(x=w268, y=w267) -> (x < y?=w266:bool)
                  }
                }
                n204 = Tick Count (ms)() -> (millisecond timer value=w255:u32)
                n205 = First Call?() -> (First Call?: T/F=w259:bool)
                n206 = case shown="True" w259 {
                  tunnel: w255 -> [w274 w280]
                  tunnel: [w270 WPI_SolenoidValue."Forward" ("Value")] -> w258
                  frame False {
                    n207 = local read "tick"() -> (w269:dbl)
                    n208 = Less Or Equal?(x=w269, y=w274) -> (x <= y?=w271:bool)
                    n209 = Select(t=WPI_SolenoidValue."Reverse" ("Value"), s=w271, f=WPI_SolenoidValue."Forward" ("Value")) -> (s? t:f=w270:T8)
                  }
                  frame True {
                    n210 = call <vilib>:"SD Read Number.vi"("Table Prefix"="SmartDashboard", "Name"="Launch Wait Time") -> ("Numeric"=w275:dbl)  [unwired: 7 in, 2 out]
                    n211 = Add(x=w280, y=w275) -> (x+y=w278:dbl)
                    n212 = local write "tick"(w278) -> ()
                  }
                }
                n213 = call <vilib>:"WPI_SolenoidRefNum Registry Get.vi"("refnum name"="Launch Cylinder") -> ("SolenoidDevRef"=w257:T20)  [unwired: 9 in, 1 out]
                n214 = call-poly <vilib>:"WPI_SolenoidSet.vi"("Value"=w258, "SolenoidDevRef"=w257) -> ()  [unwired: 8 in, 2 out]
              }
            }
          }
        }
        frame "Corner" {
          n215 = stacked-sequence {
            frame #0 {
              n216 = while {
                stop <- w281 stop-if-true
                n217 = stacked-sequence {
                  tunnel: [_ w293] -> w281
                  frame #0 {
                    n218 = local read "Numeric 0"() -> (w288:dbl)
                    n219 = Tick Count (ms)() -> (millisecond timer value=w290:u32)
                    n220 = First Call?() -> (First Call?: T/F=w291:bool)
                    n221 = Select(t=w290, s=w291, f=w288) -> (s? t:f=→"Numeric 0":dbl)
                  }
                  frame #1 {
                    n222 = local read "Numeric 0"() -> (w296:dbl)
                    n223 = Add(x="Drive wait time cr", y=w296) -> (x+y=w295:dbl)
                    n224 = Tick Count (ms)() -> (millisecond timer value=w294:u32)
                    n225 = Less?(x=w295, y=w294) -> (x < y?=w293:bool)
                  }
                }
                n226 = call <vilib>:"WPI_RobotDriveRefNum Registry Get.vi"("refnum name"="Left and Right Motors") -> ("RobotDriveDevRef"=w286:T9)  [unwired: 1 in, 9 out]
                n227 = call <vilib>:"WPI_RobotDriveArcadeDrive_Standard(NoSaturation).vi"("Y axis value"=1.0 ("X axis value"), "X axis value"=0.0, "RobotDriveDevRef"=w286) -> ("Motor Values"=w284:dbl[])  [unwired: 1 in, 7 out]
                n228 = call <vilib>:"SD Write Numeric Array.vi"("Numeric Array"=w284, "Name"="RobotDrive Motors") -> ()  [unwired: 8 in, 2 out]
              }
            }
            frame #1 {
              n229 = disable-structure shown="Disabled" {
                frame Disabled {
                  n230 = while {
                    stop <- w297 stop-if-true
                    n231 = stacked-sequence {
                      tunnel: [_ w310] -> w297
                      frame #0 {
                        n232 = local read "Numeric 0"() -> (w305:dbl)
                        n233 = Tick Count (ms)() -> (millisecond timer value=w306:u32)
                        n234 = First Call?() -> (First Call?: T/F=w307:bool)
                        n235 = Select(t=w306, s=w307, f=w305) -> (s? t:f=w304:dbl)
                        n236 = local write "Numeric 0"(w304) -> ()
                      }
                      frame #1 {
                        n237 = local read "Numeric 0"() -> (w309:dbl)
                        n238 = Add(x="Turn wait time cr", y=w309) -> (x+y=w312:dbl)
                        n239 = Tick Count (ms)() -> (millisecond timer value=w311:u32)
                        n240 = Less?(x=w312, y=w311) -> (x < y?=w310:bool)
                      }
                    }
                    n241 = call <vilib>:"WPI_RobotDriveRefNum Registry Get.vi"("refnum name"="Left and Right Motors") -> ("RobotDriveDevRef"=w299:T9)  [unwired: 1 in, 9 out]
                    n242 = call <vilib>:"WPI_RobotDriveArcadeDrive_Standard(NoSaturation).vi"("Y axis value"=0.0 ("X axis value"), "X axis value"=1.0, "RobotDriveDevRef"=w299) -> ("Motor Values"=w301:dbl[])  [unwired: 1 in, 7 out]
                    n243 = call <vilib>:"SD Write Numeric Array.vi"("Numeric Array"=w301, "Name"="RobotDrive Motors") -> ()  [unwired: 8 in, 2 out]
                  }
                }
                frame Enabled {
                }
              }
            }
            frame #2 {
              n244 = disable-structure shown="Disabled" {
                frame Disabled {
                  n245 = while {
                    stop <- w340 stop-if-true
                    n246 = global read "Robot Global Data.vi" "Target Info"() -> (w358:T17)
                    n247 = Array To Cluster(array=w358) -> (cluster=w357:T18)
                    n248 = Unbundle By Name(w357) -> ("Target Info[0]"=w356:T19, "Target Info[1]"=w351:T19, "Target Info[2]"=w350:T19, "Target Info[3]"=w349:T19)
                    n249 = Unbundle By Name(w356) -> ("Center Position"=w355:cluster{"X":dbl, "Y":dbl})  [unwired: 2 out]
                    n250 = Unbundle By Name(w351) -> ("Center Position"=w354:cluster{"X":dbl, "Y":dbl}, "Distance (ft)"=w318:dbl)  [unwired: 1 out]
                    n251 = Unbundle By Name(w350) -> ("Center Position"=w353:cluster{"X":dbl, "Y":dbl}, "Distance (ft)"=w320:dbl)  [unwired: 1 out]
                    n252 = Unbundle By Name(w349) -> ("Center Position"=w352:cluster{"X":dbl, "Y":dbl}, "Distance (ft)"=w322:dbl)  [unwired: 1 out]
                    n253 = Unbundle By Name(w355) -> ("X"=w313:dbl)  [unwired: 1 out]
                    n254 = Unbundle By Name(w354) -> ("X"=w317:dbl)  [unwired: 1 out]
                    n255 = Unbundle By Name(w353) -> ("X"=w319:dbl)  [unwired: 1 out]
                    n256 = Unbundle By Name(w352) -> ("X"=w321:dbl)  [unwired: 1 out]
                    n257 = Equal To 0?(x=w318) -> (x = 0?=w348:bool)
                    n258 = Equal To 0?(x=w320) -> (x = 0?=w347:bool)
                    n259 = Equal To 0?(x=w322) -> (x = 0?=w346:bool)
                    n260 = Select(t=1.0, s=w348, f=w317) -> (s? t:f=w329:dbl)
                    n261 = Select(t=1.0, s=w347, f=w319) -> (s? t:f=w328:dbl)
                    n262 = Select(t=1.0, s=w346, f=w321) -> (s? t:f=w342:dbl)
                    n263 = Initialize Array(0.0 ("element"), 1 ("dimension size")) -> (w324:dbl[])
                    n264 = Build Array (concatenate)(w324, w313, w317, w319, w321) -> (w314:dbl[])
                    n265 = Absolute Value(x=w313) -> (abs(x)=w336:dbl)
                    n266 = Absolute Value(x=w329) -> (abs(x)=w335:dbl)
                    n267 = Absolute Value(x=w328) -> (abs(x)=w334:dbl)
                    n268 = Absolute Value(x=w342) -> (abs(x)=w327:dbl)
                    n269 = Initialize Array(0.0 ("element"), 1 ("dimension size")) -> (w337:dbl[])
                    n270 = Build Array (concatenate)(w337, w336, w335, w334, w327) -> (w330:dbl[])
                    n271 = Sort 1D Array(array=w330) -> (sorted array=w333:dbl[])
                    n272 = Index Array(array=w333, index=0) -> (element=w331:dbl)
                    n273 = Search 1D Array(1D array=w330, element=w331) -> (index of element=w323:i32)  [unwired: 1 in]
                    n274 = Index Array(array=w314, index=w323) -> (element=w315:dbl)
                    n275 = Not Equal To 0?(x=w315) -> (x != 0?=w316:bool)
                    n276 = case shown="True" w316 {
                      tunnel: [1.0 ("output") w368] -> w341
                      tunnel: w315 -> [_ w367]
                      frame False {
                        n277 = call <vilib>:"WPI_RobotDriveRefNum Registry Get.vi"("refnum name"="Left and Right Motors") -> ("RobotDriveDevRef"=w364:T9)  [unwired: 1 in, 9 out]
                        n278 = call <vilib>:"WPI_RobotDriveArcadeDrive_Standard(NoSaturation).vi"("Y axis value"=0.0, "X axis value"=0.0, "RobotDriveDevRef"=w364) -> ("Motor Values"=w362:dbl[])  [unwired: 1 in, 7 out]
                        n279 = call <vilib>:"SD Write Numeric Array.vi"("Numeric Array"=w362, "Name"="RobotDrive Motors") -> ()  [unwired: 8 in, 2 out]
                      }
                      frame True {
                        n280 = call-poly <vilib>:"PID.vi"("PID gains"="Turn PID gains", "process variable"=w367, "setpoint"=0.0 ("process variable")) -> ("output"=w369:dbl)  [unwired: 7 in, 1 out]
                        n281 = In Range and Coerce(upper limit=0.01, x=w369, lower limit=-0.01) -> (In Range?=w371:bool)  [unwired: 1 out]
                        n282 = call <vilib>:"WPI_RobotDriveRefNum Registry Get.vi"("refnum name"="Left and Right Motors") -> ("RobotDriveDevRef"=w377:T9)  [unwired: 1 in, 9 out]
                        n283 = Select(t=0.0, s=w371, f=w369) -> (s? t:f=w368:dbl)
                        n284 = call <vilib>:"WPI_RobotDriveArcadeDrive_Standard(NoSaturation).vi"("Y axis value"=0.0, "X axis value"=w368, "RobotDriveDevRef"=w377) -> ("Motor Values"=w376:dbl[])  [unwired: 1 in, 7 out]
                        n285 = call <vilib>:"SD Write Numeric Array.vi"("Numeric Array"=w376, "Name"="RobotDrive Motors") -> ()  [unwired: 8 in, 2 out]
                      }
                    }
                    n286 = Equal To 0?(x=w341) -> (x = 0?=w340:bool)
                  }
                  n287 = while {
                    stop <- w412 stop-if-true
                    # "Ordered Position Array"
                    # "DistanceArray"
                    n288 = global read "Robot Global Data.vi" "Target Info"() -> (w428:T17)
                    n289 = Array To Cluster(array=w428) -> (cluster=w427:T18)
                    n290 = Unbundle By Name(w427) -> ("Target Info[0]"=w381:T19, "Target Info[1]"=w423:T19, "Target Info[2]"=w422:T19, "Target Info[3]"=w421:T19)
                    n291 = Unbundle By Name(w381) -> ("Center Position"=w380:cluster{"X":dbl, "Y":dbl}, "Distance (ft)"=w400:dbl)  [unwired: 1 out]
                    n292 = Unbundle By Name(w423) -> ("Center Position"=w426:cluster{"X":dbl, "Y":dbl}, "Distance (ft)"=w399:dbl)  [unwired: 1 out]
                    n293 = Unbundle By Name(w422) -> ("Center Position"=w425:cluster{"X":dbl, "Y":dbl}, "Distance (ft)"=w398:dbl)  [unwired: 1 out]
                    n294 = Unbundle By Name(w421) -> ("Center Position"=w424:cluster{"X":dbl, "Y":dbl}, "Distance (ft)"=w397:dbl)  [unwired: 1 out]
                    n295 = Initialize Array(0.0 ("element"), 1 ("dimension size")) -> (w401:dbl[])
                    n296 = Unbundle By Name(w380) -> ("X"=w385:dbl)  [unwired: 1 out]
                    n297 = Build Array (concatenate)(w401, w400, w399, w398, w397) -> (w382:dbl[])
                    n298 = Unbundle By Name(w426) -> ("X"=w386:dbl)  [unwired: 1 out]
                    n299 = Unbundle By Name(w425) -> ("X"=w391:dbl)  [unwired: 1 out]
                    n300 = Unbundle By Name(w424) -> ("X"=w389:dbl)  [unwired: 1 out]
                    n301 = Equal To 0?(x=w399) -> (x = 0?=w420:bool)
                    n302 = Equal To 0?(x=w398) -> (x = 0?=w419:bool)
                    n303 = Equal To 0?(x=w397) -> (x = 0?=w418:bool)
                    n304 = Absolute Value(x=w385) -> (abs(x)=w384:dbl)
                    n305 = Select(t=1.0, s=w420, f=w386) -> (s? t:f=w387:dbl)
                    n306 = Select(t=1.0, s=w419, f=w391) -> (s? t:f=w390:dbl)
                    n307 = Select(t=1.0, s=w418, f=w389) -> (s? t:f=w414:dbl)
                    n308 = Absolute Value(x=w387) -> (abs(x)=w408:dbl)
                    n309 = Absolute Value(x=w390) -> (abs(x)=w407:dbl)
                    n310 = Absolute Value(x=w414) -> (abs(x)=w388:dbl)
                    n311 = Initialize Array(0.0 ("element"), 1 ("dimension size")) -> (w409:dbl[])
                    n312 = Build Array (concatenate)(w409, w384, w408, w407, w388) -> (w404:dbl[])
                    n313 = Sort 1D Array(array=w404) -> (sorted array=w383:dbl[])
                    n314 = Index Array(array=w383, index=0) -> (element=w405:dbl)
                    n315 = Search 1D Array(1D array=w404, element=w405) -> (index of element=w396:i32)  [unwired: 1 in]
                    n316 = Index Array(array=w382, index=w396) -> (element=w394:dbl)
                    n317 = Subtract(x=w394, y="Sweet Spot") -> (x-y=w393:dbl)
                    n318 = Not Equal To 0?(x=w393) -> (x != 0?=w392:bool)
                    n319 = case shown="True" w392 {
                      tunnel: [1.0 ("output") w438] -> w413
                      tunnel: w393 -> [_ w439]
                      frame False {
                        n320 = call <vilib>:"WPI_RobotDriveRefNum Registry Get.vi"("refnum name"="Left and Right Motors") -> ("RobotDriveDevRef"=w434:T9)  [unwired: 1 in, 9 out]
                        n321 = call <vilib>:"WPI_RobotDriveArcadeDrive_Standard(NoSaturation).vi"("Y axis value"=0.0, "X axis value"=0.0, "RobotDriveDevRef"=w434) -> ("Motor Values"=w432:dbl[])  [unwired: 1 in, 7 out]
                        n322 = call <vilib>:"SD Write Numeric Array.vi"("Numeric Array"=w432, "Name"="RobotDrive Motors") -> ()  [unwired: 8 in, 2 out]
                      }
                      frame True {
                        n323 = local read "Drive PID gains"() -> (w436:T2)
                        n324 = call-poly <vilib>:"PID.vi"("PID gains"=w436, "process variable"=w439, "setpoint"=0.0 ("process variable")) -> ("output"=w440:dbl)  [unwired: 7 in, 1 out]
                        n325 = In Range and Coerce(upper limit=0.01, x=w440, lower limit=-0.01) -> (In Range?=w442:bool)  [unwired: 1 out]
                        n326 = call <vilib>:"WPI_RobotDriveRefNum Registry Get.vi"("refnum name"="Left and Right Motors") -> ("RobotDriveDevRef"=w447:T9)  [unwired: 1 in, 9 out]
                        n327 = Select(t=0.0, s=w442, f=w440) -> (s? t:f=w438:dbl)
                        n328 = call <vilib>:"WPI_RobotDriveArcadeDrive_Standard(NoSaturation).vi"("Y axis value"=w438, "X axis value"=0.0, "RobotDriveDevRef"=w447) -> ("Motor Values"=w446:dbl[])  [unwired: 1 in, 7 out]
                        n329 = call <vilib>:"SD Write Numeric Array.vi"("Numeric Array"=w446, "Name"="RobotDrive Motors") -> ()  [unwired: 8 in, 2 out]
                      }
                    }
                    n330 = Equal To 0?(x=w413) -> (x = 0?=w412:bool)
                  }
                }
                frame Enabled {
                }
              }
            }
            frame #3 {
              n331 = while {
                stop <- w469 stop-if-true
                # "Slow motor will always be slower"
                n332 = stacked-sequence {
                  tunnel: [_ w478] -> w469
                  frame #0 {
                    n333 = local read "Numeric 0"() -> (w474:dbl)
                    n334 = Tick Count (ms)() -> (millisecond timer value=w475:u32)
                    n335 = First Call?() -> (First Call?: T/F=w476:bool)
                    n336 = Select(t=w475, s=w476, f=w474) -> (s? t:f=w473:dbl)
                    n337 = local write "Numeric 0"(w473) -> ()
                  }
                  frame #1 {
                    n338 = local read "Launcher Charge time"() -> (w477:dbl)
                    n339 = local read "Numeric 0"() -> (w481:dbl)
                    n340 = Add(x=w477, y=w481) -> (x+y=w480:dbl)
                    n341 = Tick Count (ms)() -> (millisecond timer value=w479:u32)
                    n342 = Less?(x=w480, y=w479) -> (x < y?=w478:bool)
                  }
                }
                n343 = call <vilib>:"WPI_JoystickRefNum Registry Get.vi"("refnum name"="Joystick 1") -> ("JoystickDevRef"=w471:T5)  [unwired: 1 in, 9 out]
                n344 = call <vilib>:"WPI_JoystickGet.vi"("JoystickDevRef"=w471) -> ("Axes"=w472:T7)  [unwired: 1 in, 5 out]
                n345 = Unbundle By Name(w472) -> ("axis 3 (throttle)"=w452:dbl)
                n346 = In Range and Coerce(upper limit=1.0, x=w452, lower limit=0.0) -> (coerced(x)=w455:dbl)  [unwired: 1 out]
                n347 = Subtract(x=1.0, y=w455) -> (x-y=w466:dbl)
                n348 = In Range and Coerce(upper limit=1.0, x=w466, lower limit=0.0) -> (coerced(x)=w450:dbl)  [unwired: 1 out]
                n349 = Divide(x=w450, y="-Fast-Slow Variable") -> (x/y=w464:dbl)
                n350 = Negate(x=w450) -> (-x=w454:dbl)
                n351 = call <vilib>:"WPI_MotorControlRefNum Registry Get.vi"("refnum name"="Launch Motor Fast") -> ("error out"=w462:errorcluster, "MotorControlDevRef"=w461:T10)  [unwired: 9 in]
                n352 = call <vilib>:"WPI_MotorControlSetOutput.vi"("error in (no error)"=w462, "Output"=w454, "MotorControlDevRef"=w461) -> ()  [unwired: 6 in, 3 out]
                n353 = Negate(x=w464) -> (-x=w453:dbl)
                n354 = call <vilib>:"WPI_MotorControlRefNum Registry Get.vi"("refnum name"="Launch Motor Slow") -> ("error out"=w459:errorcluster, "MotorControlDevRef"=w460:T10)  [unwired: 9 in]
                n355 = call <vilib>:"WPI_MotorControlSetOutput.vi"("error in (no error)"=w459, "Output"=w453, "MotorControlDevRef"=w460) -> ()  [unwired: 6 in, 3 out]
              }
            }
            frame #4 {
              n356 = while {
                stop <- w482 stop-if-true
                n357 = stacked-sequence {
                  tunnel: [_ w493] -> w482
                  frame #0 {
                    n358 = local read "Numeric 0"() -> (w489:dbl)
                    n359 = Tick Count (ms)() -> (millisecond timer value=w490:u32)
                    n360 = First Call?() -> (First Call?: T/F=w491:bool)
                    n361 = Select(t=w490, s=w491, f=w489) -> (s? t:f=w488:dbl)
                    n362 = local write "Numeric 0"(w488) -> ()
                  }
                  frame #1 {
                    n363 = local read "Time between launches"() -> (w492:dbl)
                    n364 = local read "Numeric 0"() -> (w496:dbl)
                    n365 = Add(x=w492, y=w496) -> (x+y=w495:dbl)
                    n366 = Tick Count (ms)() -> (millisecond timer value=w494:u32)
                    n367 = Less?(x=w495, y=w494) -> (x < y?=w493:bool)
                  }
                }
                n368 = Tick Count (ms)() -> (millisecond timer value=w483:u32)
                n369 = First Call?() -> (First Call?: T/F=w487:bool)
                n370 = case shown="True" w487 {
                  tunnel: w483 -> [w501 w508]
                  tunnel: [w497 WPI_SolenoidValue."Forward" ("Value")] -> w486
                  frame False {
                    n371 = local read "tick"() -> (w502:dbl)
                    n372 = Less Or Equal?(x=w502, y=w501) -> (x <= y?=w498:bool)
                    n373 = Select(t=WPI_SolenoidValue."Reverse" ("Value"), s=w498, f=WPI_SolenoidValue."Forward" ("Value")) -> (s? t:f=w497:T8)
                  }
                  frame True {
                    n374 = call <vilib>:"SD Read Number.vi"("Table Prefix"="SmartDashboard", "Name"="Launch Wait Time") -> ("Numeric"=w503:dbl)  [unwired: 7 in, 2 out]
                    n375 = Add(x=w508, y=w503) -> (x+y=→"tick":dbl)
                  }
                }
                n376 = call <vilib>:"WPI_SolenoidRefNum Registry Get.vi"("refnum name"="Launch Cylinder") -> ("SolenoidDevRef"=w485:T20)  [unwired: 9 in, 1 out]
                n377 = call-poly <vilib>:"WPI_SolenoidSet.vi"("Value"=w486, "SolenoidDevRef"=w485) -> ()  [unwired: 8 in, 2 out]
              }
            }
            frame #5 {
              n378 = while {
                stop <- w509 stop-if-true
                n379 = stacked-sequence {
                  tunnel: [_ w521] -> w509
                  frame #0 {
                    n380 = local read "Numeric 0"() -> (w516:dbl)
                    n381 = Tick Count (ms)() -> (millisecond timer value=w517:u32)
                    n382 = First Call?() -> (First Call?: T/F=w518:bool)
                    n383 = Select(t=w517, s=w518, f=w516) -> (s? t:f=w515:dbl)
                    n384 = local write "Numeric 0"(w515) -> ()
                  }
                  frame #1 {
                    n385 = local read "Numeric 0"() -> (w520:dbl)
                    n386 = Add(x="Time between launches", y=w520) -> (x+y=w523:dbl)
                    n387 = Tick Count (ms)() -> (millisecond timer value=w522:u32)
                    n388 = Less?(x=w523, y=w522) -> (x < y?=w521:bool)
                  }
                }
                n389 = Tick Count (ms)() -> (millisecond timer value=w510:u32)
                n390 = First Call?() -> (First Call?: T/F=w514:bool)
                n391 = case shown="True" w514 {
                  tunnel: w510 -> [w529 w535]
                  tunnel: [w525 WPI_SolenoidValue."Forward" ("Value")] -> w513
                  frame False {
                    n392 = local read "tick"() -> (w524:dbl)
                    n393 = Less Or Equal?(x=w524, y=w529) -> (x <= y?=w526:bool)
                    n394 = Select(t=WPI_SolenoidValue."Reverse" ("Value"), s=w526, f=WPI_SolenoidValue."Forward" ("Value")) -> (s? t:f=w525:T8)
                  }
                  frame True {
                    n395 = call <vilib>:"SD Read Number.vi"("Table Prefix"="SmartDashboard", "Name"="Launch Wait Time") -> ("Numeric"=w530:dbl)  [unwired: 7 in, 2 out]
                    n396 = Add(x=w535, y=w530) -> (x+y=w533:dbl)
                    n397 = local write "tick"(w533) -> ()
                  }
                }
                n398 = call <vilib>:"WPI_SolenoidRefNum Registry Get.vi"("refnum name"="Launch Cylinder") -> ("SolenoidDevRef"=w512:T20)  [unwired: 9 in, 1 out]
                n399 = call-poly <vilib>:"WPI_SolenoidSet.vi"("Value"=w513, "SolenoidDevRef"=w512) -> ()  [unwired: 8 in, 2 out]
              }
            }
          }
        }
        frame "Corner" {
          n400 = stacked-sequence {
            frame #0 {
              n401 = while {
                stop <- w536 stop-if-true
                n402 = stacked-sequence {
                  tunnel: [_ w548] -> w536
                  frame #0 {
                    n403 = local read "Numeric 0"() -> (w544:dbl)
                    n404 = Tick Count (ms)() -> (millisecond timer value=w545:u32)
                    n405 = First Call?() -> (First Call?: T/F=w546:bool)
                    n406 = Select(t=w545, s=w546, f=w544) -> (s? t:f=w543:dbl)
                    n407 = local write "Numeric 0"(w543) -> ()
                  }
                  frame #1 {
                    n408 = local read "Numeric 0"() -> (w551:dbl)
                    n409 = Add(x="Drive wait time fl", y=w551) -> (x+y=w550:dbl)
                    n410 = Tick Count (ms)() -> (millisecond timer value=w549:u32)
                    n411 = Less?(x=w550, y=w549) -> (x < y?=w548:bool)
                  }
                }
                n412 = call <vilib>:"WPI_RobotDriveRefNum Registry Get.vi"("refnum name"="Left and Right Motors") -> ("RobotDriveDevRef"=w541:T9)  [unwired: 1 in, 9 out]
                n413 = call <vilib>:"WPI_RobotDriveArcadeDrive_Standard(NoSaturation).vi"("Y axis value"=1.0 ("X axis value"), "X axis value"=0.0, "RobotDriveDevRef"=w541) -> ("Motor Values"=w539:dbl[])  [unwired: 1 in, 7 out]
                n414 = call <vilib>:"SD Write Numeric Array.vi"("Numeric Array"=w539, "Name"="RobotDrive Motors") -> ()  [unwired: 8 in, 2 out]
              }
            }
            frame #1 {
              n415 = disable-structure shown="Disabled" {
                frame Disabled {
                  n416 = while {
                    stop <- w552 stop-if-true
                    n417 = stacked-sequence {
                      tunnel: [_ w564] -> w552
                      frame #0 {
                        n418 = local read "Numeric 0"() -> (w560:dbl)
                        n419 = Tick Count (ms)() -> (millisecond timer value=w561:u32)
                        n420 = First Call?() -> (First Call?: T/F=w562:bool)
                        n421 = Select(t=w561, s=w562, f=w560) -> (s? t:f=w559:dbl)
                        n422 = local write "Numeric 0"(w559) -> ()
                      }
                      frame #1 {
                        n423 = local read "Numeric 0"() -> (w567:dbl)
                        n424 = Add(x="Turn wait time fl", y=w567) -> (x+y=w566:dbl)
                        n425 = Tick Count (ms)() -> (millisecond timer value=w565:u32)
                        n426 = Less?(x=w566, y=w565) -> (x < y?=w564:bool)
                      }
                    }
                    n427 = call <vilib>:"WPI_RobotDriveRefNum Registry Get.vi"("refnum name"="Left and Right Motors") -> ("RobotDriveDevRef"=w554:T9)  [unwired: 1 in, 9 out]
                    n428 = call <vilib>:"WPI_RobotDriveArcadeDrive_Standard(NoSaturation).vi"("Y axis value"=0.0 ("X axis value"), "X axis value"=-1.0, "RobotDriveDevRef"=w554) -> ("Motor Values"=w556:dbl[])  [unwired: 1 in, 7 out]
                    n429 = call <vilib>:"SD Write Numeric Array.vi"("Numeric Array"=w556, "Name"="RobotDrive Motors") -> ()  [unwired: 8 in, 2 out]
                  }
                }
                frame Enabled {
                }
              }
            }
            frame #2 {
              n430 = disable-structure shown="Disabled" {
                frame Disabled {
                  n431 = while {
                    stop <- w595 stop-if-true
                    n432 = global read "Robot Global Data.vi" "Target Info"() -> (w613:T17)
                    n433 = Array To Cluster(array=w613) -> (cluster=w612:T18)
                    n434 = Unbundle By Name(w612) -> ("Target Info[0]"=w611:T19, "Target Info[1]"=w606:T19, "Target Info[2]"=w605:T19, "Target Info[3]"=w604:T19)
                    n435 = Unbundle By Name(w611) -> ("Center Position"=w610:cluster{"X":dbl, "Y":dbl})  [unwired: 2 out]
                    n436 = Unbundle By Name(w606) -> ("Center Position"=w609:cluster{"X":dbl, "Y":dbl}, "Distance (ft)"=w572:dbl)  [unwired: 1 out]
                    n437 = Unbundle By Name(w605) -> ("Center Position"=w608:cluster{"X":dbl, "Y":dbl}, "Distance (ft)"=w574:dbl)  [unwired: 1 out]
                    n438 = Unbundle By Name(w604) -> ("Center Position"=w607:cluster{"X":dbl, "Y":dbl}, "Distance (ft)"=w576:dbl)  [unwired: 1 out]
                    n439 = Unbundle By Name(w610) -> ("X"=w570:dbl)  [unwired: 1 out]
                    n440 = Unbundle By Name(w609) -> ("X"=w571:dbl)  [unwired: 1 out]
                    n441 = Unbundle By Name(w608) -> ("X"=w573:dbl)  [unwired: 1 out]
                    n442 = Unbundle By Name(w607) -> ("X"=w575:dbl)  [unwired: 1 out]
                    n443 = Equal To 0?(x=w572) -> (x = 0?=w603:bool)
                    n444 = Equal To 0?(x=w574) -> (x = 0?=w602:bool)
                    n445 = Equal To 0?(x=w576) -> (x = 0?=w601:bool)
                    n446 = Select(t=1.0, s=w603, f=w571) -> (s? t:f=w584:dbl)
                    n447 = Select(t=1.0, s=w602, f=w573) -> (s? t:f=w583:dbl)
                    n448 = Select(t=1.0, s=w601, f=w575) -> (s? t:f=w597:dbl)
                    n449 = Initialize Array(0.0 ("element"), 1 ("dimension size")) -> (w579:dbl[])
                    n450 = Build Array (concatenate)(w579, w570, w571, w573, w575) -> (w578:dbl[])
                    n451 = Absolute Value(x=w570) -> (abs(x)=w591:dbl)
                    n452 = Absolute Value(x=w584) -> (abs(x)=w590:dbl)
                    n453 = Absolute Value(x=w583) -> (abs(x)=w589:dbl)
                    n454 = Absolute Value(x=w597) -> (abs(x)=w582:dbl)
                    n455 = Initialize Array(0.0 ("element"), 1 ("dimension size")) -> (w592:dbl[])
                    n456 = Build Array (concatenate)(w592, w591, w590, w589, w582) -> (w585:dbl[])
                    n457 = Sort 1D Array(array=w585) -> (sorted array=w588:dbl[])
                    n458 = Index Array(array=w588, index=0) -> (element=w586:dbl)
                    n459 = Search 1D Array(1D array=w585, element=w586) -> (index of element=w577:i32)  [unwired: 1 in]
                    n460 = Index Array(array=w578, index=w577) -> (element=w568:dbl)
                    n461 = Not Equal To 0?(x=w568) -> (x != 0?=w569:bool)
                    n462 = case shown="True" w569 {
                      tunnel: [1.0 ("output") w623] -> w596
                      tunnel: w568 -> [_ w622]
                      frame False {
                        n463 = call <vilib>:"WPI_RobotDriveRefNum Registry Get.vi"("refnum name"="Left and Right Motors") -> ("RobotDriveDevRef"=w619:T9)  [unwired: 1 in, 9 out]
                        n464 = call <vilib>:"WPI_RobotDriveArcadeDrive_Standard(NoSaturation).vi"("Y axis value"=0.0, "X axis value"=0.0, "RobotDriveDevRef"=w619) -> ("Motor Values"=w617:dbl[])  [unwired: 1 in, 7 out]
                        n465 = call <vilib>:"SD Write Numeric Array.vi"("Numeric Array"=w617, "Name"="RobotDrive Motors") -> ()  [unwired: 8 in, 2 out]
                      }
                      frame True {
                        n466 = local read "Turn PID gains"() -> (w621:T2)
                        n467 = call-poly <vilib>:"PID.vi"("PID gains"=w621, "process variable"=w622, "setpoint"=0.0 ("process variable")) -> ("output"=w624:dbl)  [unwired: 7 in, 1 out]
                        n468 = In Range and Coerce(upper limit=0.01, x=w624, lower limit=-0.01) -> (In Range?=w626:bool)  [unwired: 1 out]
                        n469 = call <vilib>:"WPI_RobotDriveRefNum Registry Get.vi"("refnum name"="Left and Right Motors") -> ("RobotDriveDevRef"=w632:T9)  [unwired: 1 in, 9 out]
                        n470 = Select(t=0.0, s=w626, f=w624) -> (s? t:f=w623:dbl)
                        n471 = call <vilib>:"WPI_RobotDriveArcadeDrive_Standard(NoSaturation).vi"("Y axis value"=0.0, "X axis value"=w623, "RobotDriveDevRef"=w632) -> ("Motor Values"=w631:dbl[])  [unwired: 1 in, 7 out]
                        n472 = call <vilib>:"SD Write Numeric Array.vi"("Numeric Array"=w631, "Name"="RobotDrive Motors") -> ()  [unwired: 8 in, 2 out]
                      }
                    }
                    n473 = Equal To 0?(x=w596) -> (x = 0?=w595:bool)
                  }
                  n474 = while {
                    stop <- w666 stop-if-true
                    n475 = global read "Robot Global Data.vi" "Target Info"() -> (w687:T17)
                    n476 = Array To Cluster(array=w687) -> (cluster=w686:T18)
                    n477 = Unbundle By Name(w686) -> ("Target Info[0]"=w685:T19, "Target Info[1]"=w680:T19, "Target Info[2]"=w679:T19, "Target Info[3]"=w678:T19)
                    n478 = Unbundle By Name(w685) -> ("Center Position"=w684:cluster{"X":dbl, "Y":dbl}, "Distance (ft)"=w644:dbl)  [unwired: 1 out]
                    n479 = Unbundle By Name(w680) -> ("Center Position"=w683:cluster{"X":dbl, "Y":dbl}, "Distance (ft)"=w643:dbl)  [unwired: 1 out]
                    n480 = Unbundle By Name(w679) -> ("Center Position"=w682:cluster{"X":dbl, "Y":dbl}, "Distance (ft)"=w642:dbl)  [unwired: 1 out]
                    n481 = Unbundle By Name(w678) -> ("Center Position"=w681:cluster{"X":dbl, "Y":dbl}, "Distance (ft)"=w641:dbl)  [unwired: 1 out]
                    n482 = Unbundle By Name(w684) -> ("X"=w652:dbl)  [unwired: 1 out]
                    n483 = Unbundle By Name(w683) -> ("X"=w669:dbl)  [unwired: 1 out]
                    n484 = Unbundle By Name(w682) -> ("X"=w676:dbl)  [unwired: 1 out]
                    n485 = Unbundle By Name(w681) -> ("X"=w677:dbl)  [unwired: 1 out]
                    n486 = Equal To 0?(x=w643) -> (x = 0?=w675:bool)
                    n487 = Equal To 0?(x=w642) -> (x = 0?=w674:bool)
                    n488 = Equal To 0?(x=w641) -> (x = 0?=w673:bool)
                    n489 = Initialize Array(0.0 ("element"), 1 ("dimension size")) -> (w645:dbl[])
                    n490 = Build Array (concatenate)(w645, w644, w643, w642, w641) -> (w640:dbl[])
                    n491 = Select(t=1.0, s=w673, f=w677) -> (s? t:f=w668:dbl)
                    n492 = Select(t=1.0, s=w675, f=w669) -> (s? t:f=w651:dbl)
                    n493 = Select(t=1.0, s=w674, f=w676) -> (s? t:f=w650:dbl)
                    n494 = Absolute Value(x=w652) -> (abs(x)=w662:dbl)
                    n495 = Absolute Value(x=w651) -> (abs(x)=w661:dbl)
                    n496 = Absolute Value(x=w650) -> (abs(x)=w660:dbl)
                    n497 = Absolute Value(x=w668) -> (abs(x)=w649:dbl)
                    n498 = Initialize Array(0.0 ("element"), 1 ("dimension size")) -> (w663:dbl[])
                    n499 = Initialize Array(0.0 ("element"), 1 ("dimension size")) -> (w653:dbl[])
                    n500 = Build Array (concatenate)(w653, w652, w651, w650, w649) -> (w648:dbl[])
                    n501 = Build Array (concatenate)(w663, w662, w661, w660, w649) -> (w656:dbl[])
                    n502 = Sort 1D Array(array=w656) -> (sorted array=w659:dbl[])
                    n503 = Index Array(array=w659, index=0) -> (element=w657:dbl)
                    n504 = Search 1D Array(1D array=w656, element=w657) -> (index of element=w639:i32)  [unwired: 1 in]
                    n505 = local read "Sweet Spot"() -> (w635:dbl)
                    n506 = Index Array(array=w648, index=w639) -> ()  [unwired: 1 out]
                    n507 = Index Array(array=w640, index=w639) -> (element=w638:dbl)
                    n508 = Subtract(x=w638, y=w635) -> (x-y=w637:dbl)
                    n509 = Not Equal To 0?(x=w637) -> (x != 0?=w636:bool)
                    n510 = case shown="True" w636 {
                      tunnel: [1.0 ("output") w697] -> w667
                      tunnel: w637 -> [_ w698]
                      frame False {
                        n511 = call <vilib>:"WPI_RobotDriveRefNum Registry Get.vi"("refnum name"="Left and Right Motors") -> ("RobotDriveDevRef"=w693:T9)  [unwired: 1 in, 9 out]
                        n512 = call <vilib>:"WPI_RobotDriveArcadeDrive_Standard(NoSaturation).vi"("Y axis value"=0.0, "X axis value"=0.0, "RobotDriveDevRef"=w693) -> ("Motor Values"=w691:dbl[])  [unwired: 1 in, 7 out]
                        n513 = call <vilib>:"SD Write Numeric Array.vi"("Numeric Array"=w691, "Name"="RobotDrive Motors") -> ()  [unwired: 8 in, 2 out]
                      }
                      frame True {
                        n514 = local read "Drive PID gains"() -> (w695:T2)
                        n515 = call-poly <vilib>:"PID.vi"("PID gains"=w695, "process variable"=w698, "setpoint"=0.0 ("process variable")) -> ("output"=w699:dbl)  [unwired: 7 in, 1 out]
                        n516 = In Range and Coerce(upper limit=0.01, x=w699, lower limit=-0.01) -> (In Range?=w701:bool)  [unwired: 1 out]
                        n517 = call <vilib>:"WPI_RobotDriveRefNum Registry Get.vi"("refnum name"="Left and Right Motors") -> ("RobotDriveDevRef"=w706:T9)  [unwired: 1 in, 9 out]
                        n518 = Select(t=0.0, s=w701, f=w699) -> (s? t:f=w697:dbl)
                        n519 = call <vilib>:"WPI_RobotDriveArcadeDrive_Standard(NoSaturation).vi"("Y axis value"=w697, "X axis value"=0.0, "RobotDriveDevRef"=w706) -> ("Motor Values"=w705:dbl[])  [unwired: 1 in, 7 out]
                        n520 = call <vilib>:"SD Write Numeric Array.vi"("Numeric Array"=w705, "Name"="RobotDrive Motors") -> ()  [unwired: 8 in, 2 out]
                      }
                    }
                    n521 = Equal To 0?(x=w667) -> (x = 0?=w666:bool)
                  }
                }
                frame Enabled {
                }
              }
            }
            frame #3 {
              n522 = while {
                stop <- w728 stop-if-true
                # "Slow motor will always be slower"
                n523 = stacked-sequence {
                  tunnel: [_ w737] -> w728
                  frame #0 {
                    n524 = local read "Numeric 0"() -> (w733:dbl)
                    n525 = Tick Count (ms)() -> (millisecond timer value=w734:u32)
                    n526 = First Call?() -> (First Call?: T/F=w735:bool)
                    n527 = Select(t=w734, s=w735, f=w733) -> (s? t:f=w732:dbl)
                    n528 = local write "Numeric 0"(w732) -> ()
                  }
                  frame #1 {
                    n529 = local read "Launcher Charge time"() -> (w736:dbl)
                    n530 = local read "Numeric 0"() -> (w740:dbl)
                    n531 = Add(x=w736, y=w740) -> (x+y=w739:dbl)
                    n532 = Tick Count (ms)() -> (millisecond timer value=w738:u32)
                    n533 = Less?(x=w739, y=w738) -> (x < y?=w737:bool)
                  }
                }
                n534 = call <vilib>:"WPI_JoystickRefNum Registry Get.vi"("refnum name"="Joystick 1") -> ("JoystickDevRef"=w730:T5)  [unwired: 1 in, 9 out]
                n535 = call <vilib>:"WPI_JoystickGet.vi"("JoystickDevRef"=w730) -> ("Axes"=w731:T7)  [unwired: 1 in, 5 out]
                n536 = Unbundle By Name(w731) -> ("axis 3 (throttle)"=w710:dbl)
                n537 = In Range and Coerce(upper limit=1.0, x=w710, lower limit=0.0) -> (coerced(x)=w713:dbl)  [unwired: 1 out]
                n538 = Subtract(x=1.0, y=w713) -> (x-y=w725:dbl)
                n539 = local read "-Fast-Slow Variable"() -> (w709:dbl)
                n540 = In Range and Coerce(upper limit=1.0, x=w725, lower limit=0.0) -> (coerced(x)=w724:dbl)  [unwired: 1 out]
                n541 = Divide(x=w724, y=w709) -> (x/y=w722:dbl)
                n542 = Negate(x=w724) -> (-x=w712:dbl)
                n543 = call <vilib>:"WPI_MotorControlRefNum Registry Get.vi"("refnum name"="Launch Motor Fast") -> ("error out"=w720:errorcluster, "MotorControlDevRef"=w719:T10)  [unwired: 9 in]
                n544 = call <vilib>:"WPI_MotorControlSetOutput.vi"("error in (no error)"=w720, "Output"=w712, "MotorControlDevRef"=w719) -> ()  [unwired: 6 in, 3 out]
                n545 = Negate(x=w722) -> (-x=w711:dbl)
                n546 = call <vilib>:"WPI_MotorControlRefNum Registry Get.vi"("refnum name"="Launch Motor Slow") -> ("error out"=w717:errorcluster, "MotorControlDevRef"=w718:T10)  [unwired: 9 in]
                n547 = call <vilib>:"WPI_MotorControlSetOutput.vi"("error in (no error)"=w717, "Output"=w711, "MotorControlDevRef"=w718) -> ()  [unwired: 6 in, 3 out]
              }
            }
            frame #4 {
              n548 = while {
                stop <- w741 stop-if-true
                n549 = stacked-sequence {
                  tunnel: [_ w752] -> w741
                  frame #0 {
                    n550 = local read "Numeric 0"() -> (w748:dbl)
                    n551 = Tick Count (ms)() -> (millisecond timer value=w749:u32)
                    n552 = First Call?() -> (First Call?: T/F=w750:bool)
                    n553 = Select(t=w749, s=w750, f=w748) -> (s? t:f=w747:dbl)
                    n554 = local write "Numeric 0"(w747) -> ()
                  }
                  frame #1 {
                    n555 = local read "Time between launches"() -> (w751:dbl)
                    n556 = local read "Numeric 0"() -> (w755:dbl)
                    n557 = Add(x=w751, y=w755) -> (x+y=w754:dbl)
                    n558 = Tick Count (ms)() -> (millisecond timer value=w753:u32)
                    n559 = Less?(x=w754, y=w753) -> (x < y?=w752:bool)
                  }
                }
                n560 = Tick Count (ms)() -> (millisecond timer value=w742:u32)
                n561 = First Call?() -> (First Call?: T/F=w746:bool)
                n562 = case shown="True" w746 {
                  tunnel: w742 -> [w760 w767]
                  tunnel: [w756 WPI_SolenoidValue."Forward" ("Value")] -> w745
                  frame False {
                    n563 = local read "tick"() -> (w761:dbl)
                    n564 = Less Or Equal?(x=w761, y=w760) -> (x <= y?=w757:bool)
                    n565 = Select(t=WPI_SolenoidValue."Reverse" ("Value"), s=w757, f=WPI_SolenoidValue."Forward" ("Value")) -> (s? t:f=w756:T8)
                  }
                  frame True {
                    n566 = call <vilib>:"SD Read Number.vi"("Table Prefix"="SmartDashboard", "Name"="Launch Wait Time") -> ("Numeric"=w762:dbl)  [unwired: 7 in, 2 out]
                    n567 = Add(x=w767, y=w762) -> (x+y=w765:dbl)
                    n568 = local write "tick"(w765) -> ()
                  }
                }
                n569 = call <vilib>:"WPI_SolenoidRefNum Registry Get.vi"("refnum name"="Launch Cylinder") -> ("SolenoidDevRef"=w744:T20)  [unwired: 9 in, 1 out]
                n570 = call-poly <vilib>:"WPI_SolenoidSet.vi"("Value"=w745, "SolenoidDevRef"=w744) -> ()  [unwired: 8 in, 2 out]
              }
            }
            frame #5 {
              n571 = while {
                stop <- w768 stop-if-true
                n572 = stacked-sequence {
                  tunnel: [_ w780] -> w768
                  frame #0 {
                    n573 = local read "Numeric 0"() -> (w775:dbl)
                    n574 = Tick Count (ms)() -> (millisecond timer value=w776:u32)
                    n575 = First Call?() -> (First Call?: T/F=w777:bool)
                    n576 = Select(t=w776, s=w777, f=w775) -> (s? t:f=w774:dbl)
                    n577 = local write "Numeric 0"(w774) -> ()
                  }
                  frame #1 {
                    n578 = local read "Time between launches"() -> (w778:dbl)
                    n579 = local read "Numeric 0"() -> (w779:dbl)
                    n580 = Add(x=w778, y=w779) -> (x+y=w782:dbl)
                    n581 = Tick Count (ms)() -> (millisecond timer value=w781:u32)
                    n582 = Less?(x=w782, y=w781) -> (x < y?=w780:bool)
                  }
                }
                n583 = Tick Count (ms)() -> (millisecond timer value=w769:u32)
                n584 = First Call?() -> (First Call?: T/F=w773:bool)
                n585 = case shown="True" w773 {
                  tunnel: w769 -> [w788 w794]
                  tunnel: [w784 WPI_SolenoidValue."Forward" ("Value")] -> w772
                  frame False {
                    n586 = local read "tick"() -> (w783:dbl)
                    n587 = Less Or Equal?(x=w783, y=w788) -> (x <= y?=w785:bool)
                    n588 = Select(t=WPI_SolenoidValue."Reverse" ("Value"), s=w785, f=WPI_SolenoidValue."Forward" ("Value")) -> (s? t:f=w784:T8)
                  }
                  frame True {
                    n589 = call <vilib>:"SD Read Number.vi"("Table Prefix"="SmartDashboard", "Name"="Launch Wait Time") -> ("Numeric"=w789:dbl)  [unwired: 7 in, 2 out]
                    n590 = Add(x=w794, y=w789) -> (x+y=w792:dbl)
                    n591 = local write "tick"(w792) -> ()
                  }
                }
                n592 = call <vilib>:"WPI_SolenoidRefNum Registry Get.vi"("refnum name"="Launch Cylinder") -> ("SolenoidDevRef"=w771:T20)  [unwired: 9 in, 1 out]
                n593 = call-poly <vilib>:"WPI_SolenoidSet.vi"("Value"=w772, "SolenoidDevRef"=w771) -> ()  [unwired: 8 in, 2 out]
              }
            }
            frame #6 {
              n594 = while {
                stop <- w795 stop-if-true
                n595 = stacked-sequence {
                  tunnel: [_ w807] -> w795
                  frame #0 {
                    n596 = local read "Numeric 0"() -> (w802:dbl)
                    n597 = Tick Count (ms)() -> (millisecond timer value=w803:u32)
                    n598 = First Call?() -> (First Call?: T/F=w804:bool)
                    n599 = Select(t=w803, s=w804, f=w802) -> (s? t:f=w801:dbl)
                    n600 = local write "Numeric 0"(w801) -> ()
                  }
                  frame #1 {
                    n601 = local read "Time between launches"() -> (w805:dbl)
                    n602 = local read "Numeric 0"() -> (w806:dbl)
                    n603 = Add(x=w805, y=w806) -> (x+y=w809:dbl)
                    n604 = Tick Count (ms)() -> (millisecond timer value=w808:u32)
                    n605 = Less?(x=w809, y=w808) -> (x < y?=w807:bool)
                  }
                }
                n606 = Tick Count (ms)() -> (millisecond timer value=w796:u32)
                n607 = First Call?() -> (First Call?: T/F=w800:bool)
                n608 = case shown="True" w800 {
                  tunnel: w796 -> [w815 w821]
                  tunnel: [w811 WPI_SolenoidValue."Forward" ("Value")] -> w799
                  frame False {
                    n609 = local read "tick"() -> (w810:dbl)
                    n610 = Less Or Equal?(x=w810, y=w815) -> (x <= y?=w812:bool)
                    n611 = Select(t=WPI_SolenoidValue."Reverse" ("Value"), s=w812, f=WPI_SolenoidValue."Forward" ("Value")) -> (s? t:f=w811:T8)
                  }
                  frame True {
                    n612 = call <vilib>:"SD Read Number.vi"("Table Prefix"="SmartDashboard", "Name"="Launch Wait Time") -> ("Numeric"=w816:dbl)  [unwired: 7 in, 2 out]
                    n613 = Add(x=w821, y=w816) -> (x+y=w819:dbl)
                    n614 = local write "tick"(w819) -> ()
                  }
                }
                n615 = call <vilib>:"WPI_SolenoidRefNum Registry Get.vi"("refnum name"="Launch Cylinder") -> ("SolenoidDevRef"=w798:T20)  [unwired: 9 in, 1 out]
                n616 = call-poly <vilib>:"WPI_SolenoidSet.vi"("Value"=w799, "SolenoidDevRef"=w798) -> ()  [unwired: 8 in, 2 out]
              }
            }
          }
        }
        frame "Corner" {
          n617 = stacked-sequence {
            frame #0 {
              n618 = while {
                stop <- w822 stop-if-true
                n619 = stacked-sequence {
                  tunnel: [_ w835] -> w822
                  frame #0 {
                    n620 = local read "Numeric 0"() -> (w830:dbl)
                    n621 = Tick Count (ms)() -> (millisecond timer value=w831:u32)
                    n622 = First Call?() -> (First Call?: T/F=w832:bool)
                    n623 = Select(t=w831, s=w832, f=w830) -> (s? t:f=w829:dbl)
                    n624 = local write "Numeric 0"(w829) -> ()
                  }
                  frame #1 {
                    n625 = local read "Numeric 0"() -> (w834:dbl)
                    n626 = Add(x="Drive wait time fr", y=w834) -> (x+y=w837:dbl)
                    n627 = Tick Count (ms)() -> (millisecond timer value=w836:u32)
                    n628 = Less?(x=w837, y=w836) -> (x < y?=w835:bool)
                  }
                }
                n629 = call <vilib>:"WPI_RobotDriveRefNum Registry Get.vi"("refnum name"="Left and Right Motors") -> ("RobotDriveDevRef"=w827:T9)  [unwired: 1 in, 9 out]
                n630 = call <vilib>:"WPI_RobotDriveArcadeDrive_Standard(NoSaturation).vi"("Y axis value"=1.0 ("X axis value"), "X axis value"=0.0, "RobotDriveDevRef"=w827) -> ("Motor Values"=w825:dbl[])  [unwired: 1 in, 7 out]
                n631 = call <vilib>:"SD Write Numeric Array.vi"("Numeric Array"=w825, "Name"="RobotDrive Motors") -> ()  [unwired: 8 in, 2 out]
              }
            }
            frame #1 {
              n632 = disable-structure shown="Disabled" {
                frame Disabled {
                  n633 = while {
                    stop <- w838 stop-if-true
                    n634 = stacked-sequence {
                      tunnel: [_ w851] -> w838
                      frame #0 {
                        n635 = local read "Numeric 0"() -> (w846:dbl)
                        n636 = Tick Count (ms)() -> (millisecond timer value=w847:u32)
                        n637 = First Call?() -> (First Call?: T/F=w848:bool)
                        n638 = Select(t=w847, s=w848, f=w846) -> (s? t:f=w845:dbl)
                        n639 = local write "Numeric 0"(w845) -> ()
                      }
                      frame #1 {
                        n640 = local read "Numeric 0"() -> (w850:dbl)
                        n641 = Add(x="Turn wait time fr", y=w850) -> (x+y=w853:dbl)
                        n642 = Tick Count (ms)() -> (millisecond timer value=w852:u32)
                        n643 = Less?(x=w853, y=w852) -> (x < y?=w851:bool)
                      }
                    }
                    n644 = call <vilib>:"WPI_RobotDriveRefNum Registry Get.vi"("refnum name"="Left and Right Motors") -> ("RobotDriveDevRef"=w840:T9)  [unwired: 1 in, 9 out]
                    n645 = call <vilib>:"WPI_RobotDriveArcadeDrive_Standard(NoSaturation).vi"("Y axis value"=0.0 ("X axis value"), "X axis value"=1.0, "RobotDriveDevRef"=w840) -> ("Motor Values"=w842:dbl[])  [unwired: 1 in, 7 out]
                    n646 = call <vilib>:"SD Write Numeric Array.vi"("Numeric Array"=w842, "Name"="RobotDrive Motors") -> ()  [unwired: 8 in, 2 out]
                  }
                }
                frame Enabled {
                }
              }
            }
            frame #2 {
              n647 = disable-structure shown="Disabled" {
                frame Disabled {
                  n648 = while {
                    stop <- w881 stop-if-true
                    n649 = global read "Robot Global Data.vi" "Target Info"() -> (w899:T17)
                    n650 = Array To Cluster(array=w899) -> (cluster=w898:T18)
                    n651 = Unbundle By Name(w898) -> ("Target Info[0]"=w897:T19, "Target Info[1]"=w892:T19, "Target Info[2]"=w891:T19, "Target Info[3]"=w890:T19)
                    n652 = Unbundle By Name(w897) -> ("Center Position"=w896:cluster{"X":dbl, "Y":dbl})  [unwired: 2 out]
                    n653 = Unbundle By Name(w892) -> ("Center Position"=w895:cluster{"X":dbl, "Y":dbl}, "Distance (ft)"=w858:dbl)  [unwired: 1 out]
                    n654 = Unbundle By Name(w891) -> ("Center Position"=w894:cluster{"X":dbl, "Y":dbl}, "Distance (ft)"=w860:dbl)  [unwired: 1 out]
                    n655 = Unbundle By Name(w890) -> ("Center Position"=w893:cluster{"X":dbl, "Y":dbl}, "Distance (ft)"=w862:dbl)  [unwired: 1 out]
                    n656 = Unbundle By Name(w896) -> ("X"=w856:dbl)  [unwired: 1 out]
                    n657 = Unbundle By Name(w895) -> ("X"=w857:dbl)  [unwired: 1 out]
                    n658 = Unbundle By Name(w894) -> ("X"=w859:dbl)  [unwired: 1 out]
                    n659 = Unbundle By Name(w893) -> ("X"=w861:dbl)  [unwired: 1 out]
                    n660 = Equal To 0?(x=w858) -> (x = 0?=w889:bool)
                    n661 = Equal To 0?(x=w860) -> (x = 0?=w888:bool)
                    n662 = Equal To 0?(x=w862) -> (x = 0?=w887:bool)
                    n663 = Select(t=1.0, s=w889, f=w857) -> (s? t:f=w870:dbl)
                    n664 = Select(t=1.0, s=w888, f=w859) -> (s? t:f=w869:dbl)
                    n665 = Select(t=1.0, s=w887, f=w861) -> (s? t:f=w883:dbl)
                    n666 = Initialize Array(0.0 ("element"), 1 ("dimension size")) -> (w865:dbl[])
                    n667 = Build Array (concatenate)(w865, w856, w857, w859, w861) -> (w864:dbl[])
                    n668 = Absolute Value(x=w856) -> (abs(x)=w877:dbl)
                    n669 = Absolute Value(x=w870) -> (abs(x)=w876:dbl)
                    n670 = Absolute Value(x=w869) -> (abs(x)=w875:dbl)
                    n671 = Absolute Value(x=w883) -> (abs(x)=w868:dbl)
                    n672 = Initialize Array(0.0 ("element"), 1 ("dimension size")) -> (w878:dbl[])
                    n673 = Build Array (concatenate)(w878, w877, w876, w875, w868) -> (w871:dbl[])
                    n674 = Sort 1D Array(array=w871) -> (sorted array=w874:dbl[])
                    n675 = Index Array(array=w874, index=0) -> (element=w872:dbl)
                    n676 = Search 1D Array(1D array=w871, element=w872) -> (index of element=w863:i32)  [unwired: 1 in]
                    n677 = Index Array(array=w864, index=w863) -> (element=w854:dbl)
                    n678 = Not Equal To 0?(x=w854) -> (x != 0?=w855:bool)
                    n679 = case shown="True" w855 {
                      tunnel: [1.0 ("output") w909] -> w882
                      tunnel: w854 -> [_ w908]
                      frame False {
                        n680 = call <vilib>:"WPI_RobotDriveRefNum Registry Get.vi"("refnum name"="Left and Right Motors") -> ("RobotDriveDevRef"=w905:T9)  [unwired: 1 in, 9 out]
                        n681 = call <vilib>:"WPI_RobotDriveArcadeDrive_Standard(NoSaturation).vi"("Y axis value"=0.0, "X axis value"=0.0, "RobotDriveDevRef"=w905) -> ("Motor Values"=w903:dbl[])  [unwired: 1 in, 7 out]
                        n682 = call <vilib>:"SD Write Numeric Array.vi"("Numeric Array"=w903, "Name"="RobotDrive Motors") -> ()  [unwired: 8 in, 2 out]
                      }
                      frame True {
                        n683 = local read "Turn PID gains"() -> (w907:T2)
                        n684 = call-poly <vilib>:"PID.vi"("PID gains"=w907, "process variable"=w908, "setpoint"=0.0 ("process variable")) -> ("output"=w910:dbl)  [unwired: 7 in, 1 out]
                        n685 = In Range and Coerce(upper limit=0.01, x=w910, lower limit=-0.01) -> (In Range?=w912:bool)  [unwired: 1 out]
                        n686 = call <vilib>:"WPI_RobotDriveRefNum Registry Get.vi"("refnum name"="Left and Right Motors") -> ("RobotDriveDevRef"=w918:T9)  [unwired: 1 in, 9 out]
                        n687 = Select(t=0.0, s=w912, f=w910) -> (s? t:f=w909:dbl)
                        n688 = call <vilib>:"WPI_RobotDriveArcadeDrive_Standard(NoSaturation).vi"("Y axis value"=0.0, "X axis value"=w909, "RobotDriveDevRef"=w918) -> ("Motor Values"=w917:dbl[])  [unwired: 1 in, 7 out]
                        n689 = call <vilib>:"SD Write Numeric Array.vi"("Numeric Array"=w917, "Name"="RobotDrive Motors") -> ()  [unwired: 8 in, 2 out]
                      }
                    }
                    n690 = Equal To 0?(x=w882) -> (x = 0?=w881:bool)
                  }
                  n691 = while {
                    stop <- w952 stop-if-true
                    n692 = global read "Robot Global Data.vi" "Target Info"() -> (w973:T17)
                    n693 = Array To Cluster(array=w973) -> (cluster=w972:T18)
                    n694 = Unbundle By Name(w972) -> ("Target Info[0]"=w971:T19, "Target Info[1]"=w966:T19, "Target Info[2]"=w965:T19, "Target Info[3]"=w964:T19)
                    n695 = Unbundle By Name(w971) -> ("Center Position"=w970:cluster{"X":dbl, "Y":dbl}, "Distance (ft)"=w930:dbl)  [unwired: 1 out]
                    n696 = Unbundle By Name(w966) -> ("Center Position"=w969:cluster{"X":dbl, "Y":dbl}, "Distance (ft)"=w929:dbl)  [unwired: 1 out]
                    n697 = Unbundle By Name(w965) -> ("Center Position"=w968:cluster{"X":dbl, "Y":dbl}, "Distance (ft)"=w928:dbl)  [unwired: 1 out]
                    n698 = Unbundle By Name(w964) -> ("Center Position"=w967:cluster{"X":dbl, "Y":dbl}, "Distance (ft)"=w927:dbl)  [unwired: 1 out]
                    n699 = Unbundle By Name(w970) -> ("X"=w938:dbl)  [unwired: 1 out]
                    n700 = Unbundle By Name(w969) -> ("X"=w955:dbl)  [unwired: 1 out]
                    n701 = Unbundle By Name(w968) -> ("X"=w962:dbl)  [unwired: 1 out]
                    n702 = Unbundle By Name(w967) -> ("X"=w963:dbl)  [unwired: 1 out]
                    n703 = Equal To 0?(x=w929) -> (x = 0?=w961:bool)
                    n704 = Equal To 0?(x=w928) -> (x = 0?=w960:bool)
                    n705 = Equal To 0?(x=w927) -> (x = 0?=w959:bool)
                    n706 = Initialize Array(0.0 ("element"), 1 ("dimension size")) -> (w931:dbl[])
                    n707 = Build Array (concatenate)(w931, w930, w929, w928, w927) -> (w926:dbl[])
                    n708 = Select(t=1.0, s=w959, f=w963) -> (s? t:f=w954:dbl)
                    n709 = Select(t=1.0, s=w961, f=w955) -> (s? t:f=w937:dbl)
                    n710 = Select(t=1.0, s=w960, f=w962) -> (s? t:f=w936:dbl)
                    n711 = Absolute Value(x=w938) -> (abs(x)=w948:dbl)
                    n712 = Absolute Value(x=w937) -> (abs(x)=w947:dbl)
                    n713 = Absolute Value(x=w936) -> (abs(x)=w946:dbl)
                    n714 = Absolute Value(x=w954) -> (abs(x)=w935:dbl)
                    n715 = Initialize Array(0.0 ("element"), 1 ("dimension size")) -> (w949:dbl[])
                    n716 = Initialize Array(0.0 ("element"), 1 ("dimension size")) -> (w939:dbl[])
                    n717 = Build Array (concatenate)(w939, w938, w937, w936, w935) -> (w934:dbl[])
                    n718 = Build Array (concatenate)(w949, w948, w947, w946, w935) -> (w942:dbl[])
                    n719 = Sort 1D Array(array=w942) -> (sorted array=w945:dbl[])
                    n720 = Index Array(array=w945, index=0) -> (element=w943:dbl)
                    n721 = Search 1D Array(1D array=w942, element=w943) -> (index of element=w925:i32)  [unwired: 1 in]
                    n722 = local read "Sweet Spot"() -> (w921:dbl)
                    n723 = Index Array(array=w934, index=w925) -> ()  [unwired: 1 out]
                    n724 = Index Array(array=w926, index=w925) -> (element=w924:dbl)
                    n725 = Subtract(x=w924, y=w921) -> (x-y=w923:dbl)
                    n726 = Not Equal To 0?(x=w923) -> (x != 0?=w922:bool)
                    n727 = case shown="True" w922 {
                      tunnel: [1.0 ("output") w983] -> w953
                      tunnel: w923 -> [_ w984]
                      frame False {
                        n728 = call <vilib>:"WPI_RobotDriveRefNum Registry Get.vi"("refnum name"="Left and Right Motors") -> ("RobotDriveDevRef"=w979:T9)  [unwired: 1 in, 9 out]
                        n729 = call <vilib>:"WPI_RobotDriveArcadeDrive_Standard(NoSaturation).vi"("Y axis value"=0.0, "X axis value"=0.0, "RobotDriveDevRef"=w979) -> ("Motor Values"=w977:dbl[])  [unwired: 1 in, 7 out]
                        n730 = call <vilib>:"SD Write Numeric Array.vi"("Numeric Array"=w977, "Name"="RobotDrive Motors") -> ()  [unwired: 8 in, 2 out]
                      }
                      frame True {
                        n731 = local read "Drive PID gains"() -> (w981:T2)
                        n732 = call-poly <vilib>:"PID.vi"("PID gains"=w981, "process variable"=w984, "setpoint"=0.0 ("process variable")) -> ("output"=w985:dbl)  [unwired: 7 in, 1 out]
                        n733 = In Range and Coerce(upper limit=0.01, x=w985, lower limit=-0.01) -> (In Range?=w987:bool)  [unwired: 1 out]
                        n734 = call <vilib>:"WPI_RobotDriveRefNum Registry Get.vi"("refnum name"="Left and Right Motors") -> ("RobotDriveDevRef"=w992:T9)  [unwired: 1 in, 9 out]
                        n735 = Select(t=0.0, s=w987, f=w985) -> (s? t:f=w983:dbl)
                        n736 = call <vilib>:"WPI_RobotDriveArcadeDrive_Standard(NoSaturation).vi"("Y axis value"=w983, "X axis value"=0.0, "RobotDriveDevRef"=w992) -> ("Motor Values"=w991:dbl[])  [unwired: 1 in, 7 out]
                        n737 = call <vilib>:"SD Write Numeric Array.vi"("Numeric Array"=w991, "Name"="RobotDrive Motors") -> ()  [unwired: 8 in, 2 out]
                      }
                    }
                    n738 = Equal To 0?(x=w953) -> (x = 0?=w952:bool)
                  }
                }
                frame Enabled {
                }
              }
            }
            frame #3 {
              n739 = while {
                stop <- w1002 stop-if-true
                n740 = stacked-sequence {
                  tunnel: [_ w1024] -> w1002
                  frame #0 {
                    n741 = local read "Numeric 0"() -> (w1019:dbl)
                    n742 = Tick Count (ms)() -> (millisecond timer value=w1020:u32)
                    n743 = First Call?() -> (First Call?: T/F=w1021:bool)
                    n744 = Select(t=w1020, s=w1021, f=w1019) -> (s? t:f=w1018:dbl)
                    n745 = local write "Numeric 0"(w1018) -> ()
                  }
                  frame #1 {
                    n746 = local read "Launcher Charge time"() -> (w1022:dbl)
                    n747 = local read "Numeric 0"() -> (w1023:dbl)
                    n748 = Add(x=w1022, y=w1023) -> (x+y=w1026:dbl)
                    n749 = Tick Count (ms)() -> (millisecond timer value=w1025:u32)
                    n750 = Less?(x=w1026, y=w1025) -> (x < y?=w1024:bool)
                  }
                }
                n751 = call <vilib>:"WPI_JoystickRefNum Registry Get.vi"("refnum name"="Joystick 1") -> ("JoystickDevRef"=w1016:T5)  [unwired: 1 in, 9 out]
                n752 = call <vilib>:"WPI_JoystickGet.vi"("JoystickDevRef"=w1016) -> ("Axes"=w1017:T7)  [unwired: 1 in, 5 out]
                n753 = Unbundle By Name(w1017) -> ("axis 3 (throttle)"=w998:dbl)
                n754 = In Range and Coerce(upper limit=1.0, x=w998, lower limit=0.0) -> (coerced(x)=w997:dbl)  [unwired: 1 out]
                n755 = Subtract(x=1.0, y=w997) -> (x-y=w1012:dbl)
                n756 = local read "-Fast-Slow Variable"() -> (w1001:dbl)
                n757 = In Range and Coerce(upper limit=1.0, x=w1012, lower limit=0.0) -> (coerced(x)=w1011:dbl)  [unwired: 1 out]
                n758 = Divide(x=w1011, y=w1001) -> (x/y=w1009:dbl)
                n759 = Negate(x=w1011) -> (-x=w996:dbl)
                n760 = call <vilib>:"WPI_MotorControlRefNum Registry Get.vi"("refnum name"="Launch Motor Fast") -> ("error out"=w1007:errorcluster, "MotorControlDevRef"=w1006:T10)  [unwired: 9 in]
                n761 = call <vilib>:"WPI_MotorControlSetOutput.vi"("error in (no error)"=w1007, "Output"=w996, "MotorControlDevRef"=w1006) -> ()  [unwired: 6 in, 3 out]
                n762 = Negate(x=w1009) -> (-x=w995:dbl)
                n763 = call <vilib>:"WPI_MotorControlRefNum Registry Get.vi"("refnum name"="Launch Motor Slow") -> ("error out"=w1004:errorcluster, "MotorControlDevRef"=w1005:T10)  [unwired: 9 in]
                n764 = call <vilib>:"WPI_MotorControlSetOutput.vi"("error in (no error)"=w1004, "Output"=w995, "MotorControlDevRef"=w1005) -> ()  [unwired: 6 in, 3 out]
              }
            }
            frame #4 {
              n765 = while {
                stop <- w1027 stop-if-true
                n766 = stacked-sequence {
                  tunnel: [_ w1039] -> w1027
                  frame #0 {
                    n767 = local read "Numeric 0"() -> (w1034:dbl)
                    n768 = Tick Count (ms)() -> (millisecond timer value=w1035:u32)
                    n769 = First Call?() -> (First Call?: T/F=w1036:bool)
                    n770 = Select(t=w1035, s=w1036, f=w1034) -> (s? t:f=w1033:dbl)
                    n771 = local write "Numeric 0"(w1033) -> ()
                  }
                  frame #1 {
                    n772 = local read "Time between launches"() -> (w1037:dbl)
                    n773 = local read "Numeric 0"() -> (w1038:dbl)
                    n774 = Add(x=w1037, y=w1038) -> (x+y=w1041:dbl)
                    n775 = Tick Count (ms)() -> (millisecond timer value=w1040:u32)
                    n776 = Less?(x=w1041, y=w1040) -> (x < y?=w1039:bool)
                  }
                }
                n777 = Tick Count (ms)() -> (millisecond timer value=w1028:u32)
                n778 = First Call?() -> (First Call?: T/F=w1032:bool)
                n779 = case shown="True" w1032 {
                  tunnel: w1028 -> [w1046 w1053]
                  tunnel: [w1042 WPI_SolenoidValue."Forward" ("Value")] -> w1031
                  frame False {
                    n780 = local read "tick"() -> (w1047:dbl)
                    n781 = Less Or Equal?(x=w1047, y=w1046) -> (x <= y?=w1043:bool)
                    n782 = Select(t=WPI_SolenoidValue."Reverse" ("Value"), s=w1043, f=WPI_SolenoidValue."Forward" ("Value")) -> (s? t:f=w1042:T8)
                  }
                  frame True {
                    n783 = call <vilib>:"SD Read Number.vi"("Table Prefix"="SmartDashboard", "Name"="Launch Wait Time") -> ("Numeric"=w1048:dbl)  [unwired: 7 in, 2 out]
                    n784 = Add(x=w1053, y=w1048) -> (x+y=w1051:dbl)
                    n785 = local write "tick"(w1051) -> ()
                  }
                }
                n786 = call <vilib>:"WPI_SolenoidRefNum Registry Get.vi"("refnum name"="Launch Cylinder") -> ("SolenoidDevRef"=w1030:T20)  [unwired: 9 in, 1 out]
                n787 = call-poly <vilib>:"WPI_SolenoidSet.vi"("Value"=w1031, "SolenoidDevRef"=w1030) -> ()  [unwired: 8 in, 2 out]
              }
            }
            frame #5 {
              n788 = while {
                stop <- w1054 stop-if-true
                n789 = stacked-sequence {
                  tunnel: [_ w1066] -> w1054
                  frame #0 {
                    n790 = local read "Numeric 0"() -> (w1061:dbl)
                    n791 = Tick Count (ms)() -> (millisecond timer value=w1062:u32)
                    n792 = First Call?() -> (First Call?: T/F=w1063:bool)
                    n793 = Select(t=w1062, s=w1063, f=w1061) -> (s? t:f=w1060:dbl)
                    n794 = local write "Numeric 0"(w1060) -> ()
                  }
                  frame #1 {
                    n795 = local read "Time between launches"() -> (w1064:dbl)
                    n796 = local read "Numeric 0"() -> (w1065:dbl)
                    n797 = Add(x=w1064, y=w1065) -> (x+y=w1068:dbl)
                    n798 = Tick Count (ms)() -> (millisecond timer value=w1067:u32)
                    n799 = Less?(x=w1068, y=w1067) -> (x < y?=w1066:bool)
                  }
                }
                n800 = Tick Count (ms)() -> (millisecond timer value=w1055:u32)
                n801 = First Call?() -> (First Call?: T/F=w1059:bool)
                n802 = case shown="True" w1059 {
                  tunnel: w1055 -> [w1074 w1080]
                  tunnel: [w1070 WPI_SolenoidValue."Forward" ("Value")] -> w1058
                  frame False {
                    n803 = local read "tick"() -> (w1069:dbl)
                    n804 = Less Or Equal?(x=w1069, y=w1074) -> (x <= y?=w1071:bool)
                    n805 = Select(t=WPI_SolenoidValue."Reverse" ("Value"), s=w1071, f=WPI_SolenoidValue."Forward" ("Value")) -> (s? t:f=w1070:T8)
                  }
                  frame True {
                    n806 = call <vilib>:"SD Read Number.vi"("Table Prefix"="SmartDashboard", "Name"="Launch Wait Time") -> ("Numeric"=w1075:dbl)  [unwired: 7 in, 2 out]
                    n807 = Add(x=w1080, y=w1075) -> (x+y=w1078:dbl)
                    n808 = local write "tick"(w1078) -> ()
                  }
                }
                n809 = call <vilib>:"WPI_SolenoidRefNum Registry Get.vi"("refnum name"="Launch Cylinder") -> ("SolenoidDevRef"=w1057:T20)  [unwired: 9 in, 1 out]
                n810 = call-poly <vilib>:"WPI_SolenoidSet.vi"("Value"=w1058, "SolenoidDevRef"=w1057) -> ()  [unwired: 8 in, 2 out]
              }
            }
            frame #6 {
              n811 = while {
                stop <- w1081 stop-if-true
                n812 = stacked-sequence {
                  tunnel: [_ w1093] -> w1081
                  frame #0 {
                    n813 = local read "Numeric 0"() -> (w1088:dbl)
                    n814 = Tick Count (ms)() -> (millisecond timer value=w1089:u32)
                    n815 = First Call?() -> (First Call?: T/F=w1090:bool)
                    n816 = Select(t=w1089, s=w1090, f=w1088) -> (s? t:f=w1087:dbl)
                    n817 = local write "Numeric 0"(w1087) -> ()
                  }
                  frame #1 {
                    n818 = local read "Time between launches"() -> (w1091:dbl)
                    n819 = local read "Numeric 0"() -> (w1092:dbl)
                    n820 = Add(x=w1091, y=w1092) -> (x+y=w1095:dbl)
                    n821 = Tick Count (ms)() -> (millisecond timer value=w1094:u32)
                    n822 = Less?(x=w1095, y=w1094) -> (x < y?=w1093:bool)
                  }
                }
                n823 = Tick Count (ms)() -> (millisecond timer value=w1082:u32)
                n824 = First Call?() -> (First Call?: T/F=w1086:bool)
                n825 = case shown="True" w1086 {
                  tunnel: w1082 -> [w1101 w1107]
                  tunnel: [w1097 WPI_SolenoidValue."Forward" ("Value")] -> w1085
                  frame False {
                    n826 = local read "tick"() -> (w1096:dbl)
                    n827 = Less Or Equal?(x=w1096, y=w1101) -> (x <= y?=w1098:bool)
                    n828 = Select(t=WPI_SolenoidValue."Reverse" ("Value"), s=w1098, f=WPI_SolenoidValue."Forward" ("Value")) -> (s? t:f=w1097:T8)
                  }
                  frame True {
                    n829 = call <vilib>:"SD Read Number.vi"("Table Prefix"="SmartDashboard", "Name"="Launch Wait Time") -> ("Numeric"=w1102:dbl)  [unwired: 7 in, 2 out]
                    n830 = Add(x=w1107, y=w1102) -> (x+y=w1105:dbl)
                    n831 = local write "tick"(w1105) -> ()
                  }
                }
                n832 = call <vilib>:"WPI_SolenoidRefNum Registry Get.vi"("refnum name"="Launch Cylinder") -> ("SolenoidDevRef"=w1084:T20)  [unwired: 9 in, 1 out]
                n833 = call-poly <vilib>:"WPI_SolenoidSet.vi"("Value"=w1085, "SolenoidDevRef"=w1084) -> ()  [unwired: 8 in, 2 out]
              }
            }
          }
        }
      }
    }
    frame Enabled {
      n834 = case shown="\"Middle\"" w1108 {
        frame "Corner" {
          n835 = flat-sequence {
            frame #0 {
              n836 = while {
                stop <- w1109 stop-if-true
                n837 = stacked-sequence {
                  tunnel: [_ w1121] -> w1109
                  frame #0 {
                    n838 = local read "Numeric 0"() -> (w1117:dbl)
                    n839 = Tick Count (ms)() -> (millisecond timer value=w1118:u32)
                    n840 = First Call?() -> (First Call?: T/F=w1119:bool)
                    n841 = Select(t=w1118, s=w1119, f=w1117) -> (s? t:f=w1116:dbl)
                    n842 = local write "Numeric 0"(w1116) -> ()
                  }
                  frame #1 {
                    n843 = local read "Drive wait time cl"() -> (w1120:dbl)
                    n844 = local read "Numeric 0"() -> (w1124:dbl)
                    n845 = Add(x=w1120, y=w1124) -> (x+y=w1123:dbl)
                    n846 = Tick Count (ms)() -> (millisecond timer value=w1122:u32)
                    n847 = Less?(x=w1123, y=w1122) -> (x < y?=w1121:bool)
                  }
                }
                n848 = call <vilib>:"WPI_RobotDriveRefNum Registry Get.vi"("refnum name"="Left and Right Motors") -> ("RobotDriveDevRef"=w1114:T9)  [unwired: 1 in, 9 out]
                n849 = call <vilib>:"WPI_RobotDriveArcadeDrive_Standard(NoSaturation).vi"("Y axis value"=1.0 ("X axis value"), "X axis value"=0.0, "RobotDriveDevRef"=w1114) -> ("Motor Values"=w1112:dbl[])  [unwired: 1 in, 7 out]
                n850 = call <vilib>:"SD Write Numeric Array.vi"("Numeric Array"=w1112, "Name"="RobotDrive Motors") -> ()  [unwired: 8 in, 2 out]
              }
            }
            frame #1 {
              n851 = Tick Count (ms)() -> (millisecond timer value=w1128:u32)
              n852 = Add(x=w1128, y="Charge Up Time") -> (x+y=→"Charge Up tick":dbl)
              n853 = Add(x=w1128, y="Launch Wait Time") -> (x+y=→"Launch Wait tick":dbl)
              n854 = Add(x=w1128, y="Time Between Launches") -> (x+y=→"Time Between tick":dbl)
            }
            frame #2 {
              n855 = while {
                stop <- FALSE stop-if-true
                n856 = case shown="\"Charge Up \"" "Quicklaunch State" {
                  frame "Charge Up " {
                    n857 = local read "Charge Up tick"() -> (w1150:dbl)
                    n858 = Tick Count (ms)() -> (millisecond timer value=w1154:u32)
                    n859 = Less Or Equal?(x=w1150, y=w1154) -> (x <= y?=w1153:bool)
                    n860 = Select(t=T1."Fire 1", s=w1153, f=T1."Charge Up ") -> (s? t:f=w1155:T1)
                    n861 = local write "Quicklaunch State"(w1155) -> ()
                  }
                  frame "Fire 1" {
                    n862 = local read "Launch Wait tick"() -> (w1164:dbl)
                    n863 = local read "Charge Up Time"() -> (w1162:dbl)
                    n864 = Add(x=w1164, y=w1162) -> (x+y=w1163:dbl)
                    n865 = Tick Count (ms)() -> (millisecond timer value=w1168:u32)
                    n866 = Less Or Equal?(x=w1163, y=w1168) -> (x <= y?=w1159:bool)
                    n867 = Select(t=WPI_SolenoidValue."Reverse" ("Value"), s=w1159, f=WPI_SolenoidValue."Forward" ("Value")) -> (s? t:f=w1156:T8)
                    n868 = call <vilib>:"WPI_SolenoidRefNum Registry Get.vi"("refnum name"="Launch Cylinder") -> ("SolenoidDevRef"=w1161:T20)  [unwired: 9 in, 1 out]
                    n869 = call-poly <vilib>:"WPI_SolenoidSet.vi"("Value"=w1156, "SolenoidDevRef"=w1161) -> ()  [unwired: 8 in, 2 out]
                    n870 = Select(t=T1."wait1", s=w1159, f=T1."Fire 1") -> (s? t:f=w1167:T1)
                    n871 = local write "Quicklaunch State"(w1167) -> ()
                  }
                  frame "wait1" {
                    n872 = local read "Time Between tick"() -> (w1170:dbl)
                    n873 = local read "Launch Wait Time"() -> (w1171:dbl)
                    n874 = local read "Charge Up Time"() -> (w1172:dbl)
                    n875 = Compound Arithmetic op=ADD(w1170, w1172, w1171) -> (w1169:dbl)
                    n876 = Tick Count (ms)() -> (millisecond timer value=w1174:u32)
                    n877 = Less Or Equal?(x=w1169, y=w1174) -> (x <= y?=w1173:bool)
                    n878 = Select(t=T1."Fire 2", s=w1173, f=T1."wait1") -> (s? t:f=w1177:T1)
                    n879 = local write "Quicklaunch State"(w1177) -> ()
                  }
                  frame "Fire 2" {
                    n880 = local read "Time Between Launches"() -> (w1179:dbl)
                    n881 = local read "Launch Wait Time"() -> (w1180:dbl)
                    n882 = local read "Launch Wait tick"() -> (w1182:dbl)
                    n883 = local read "Charge Up Time"() -> (w1181:dbl)
                    n884 = Compound Arithmetic op=ADD(w1182, w1181, w1180, w1179) -> (w1178:dbl)
                    n885 = Tick Count (ms)() -> (millisecond timer value=w1192:u32)
                    n886 = Less Or Equal?(x=w1178, y=w1192) -> (x <= y?=w1186:bool)
                    n887 = Select(t=WPI_SolenoidValue."Reverse" ("Value"), s=w1186, f=WPI_SolenoidValue."Forward" ("Value")) -> (s? t:f=w1183:T8)
                    n888 = call <vilib>:"WPI_SolenoidRefNum Registry Get.vi"("refnum name"="Launch Cylinder") -> ("SolenoidDevRef"=w1188:T20)  [unwired: 9 in, 1 out]
                    n889 = call-poly <vilib>:"WPI_SolenoidSet.vi"("Value"=w1183, "SolenoidDevRef"=w1188) -> ()  [unwired: 8 in, 2 out]
                    n890 = Select(t=T1."wait2", s=w1186, f=T1."Fire 2") -> (s? t:f=w1191:T1)
                    n891 = local write "Quicklaunch State"(w1191) -> ()
                  }
                  frame "wait2" {
                    n892 = local read "Launch Wait Time"() -> (w1198:dbl)
                    n893 = local read "Time Between Launches"() -> (w1195:dbl)
                    n894 = local read "Time Between tick"() -> (w1197:dbl)
                    n895 = local read "Charge Up Time"() -> (w1199:dbl)
                    n896 = Multiply(x=2.0, y=w1198) -> (x*y=w1194:dbl)
                    n897 = Compound Arithmetic op=ADD(w1197, w1199, w1194, w1195) -> (w1196:dbl)
                    n898 = Tick Count (ms)() -> (millisecond timer value=w1201:u32)
                    n899 = Less Or Equal?(x=w1196, y=w1201) -> (x <= y?=w1200:bool)
                    n900 = Select(t=T1."Fire 3", s=w1200, f=T1."wait2") -> (s? t:f=w1204:T1)
                    n901 = local write "Quicklaunch State"(w1204) -> ()
                  }
                  frame "Fire 3" {
                    w1205 = 2.0 ("y")
                    n902 = local read "Time Between Launches"() -> (w1208:dbl)
                    n903 = local read "Launch Wait Time"() -> (w1209:dbl)
                    n904 = local read "Launch Wait tick"() -> (w1212:dbl)
                    n905 = local read "Charge Up Time"() -> (w1211:dbl)
                    n906 = Multiply(x=w1209, y=w1205) -> (x*y=w1206:dbl)
                    n907 = Multiply(x=w1208, y=w1205) -> (x*y=w1207:dbl)
                    n908 = Compound Arithmetic op=ADD(w1212, w1211, w1206, w1207) -> (w1210:dbl)
                    n909 = Tick Count (ms)() -> (millisecond timer value=w1222:u32)
                    n910 = Less Or Equal?(x=w1210, y=w1222) -> (x <= y?=w1216:bool)
                    n911 = Select(t=WPI_SolenoidValue."Reverse" ("Value"), s=w1216, f=WPI_SolenoidValue."Forward" ("Value")) -> (s? t:f=w1213:T8)
                    n912 = call <vilib>:"WPI_SolenoidRefNum Registry Get.vi"("refnum name"="Launch Cylinder") -> ("SolenoidDevRef"=w1218:T20)  [unwired: 9 in, 1 out]
                    n913 = call-poly <vilib>:"WPI_SolenoidSet.vi"("Value"=w1213, "SolenoidDevRef"=w1218) -> ()  [unwired: 8 in, 2 out]
                    n914 = Select(t=T1."wait3", s=w1216, f=T1."Fire 3") -> (s? t:f=w1221:T1)
                    n915 = local write "Quicklaunch State"(w1221) -> ()
                  }
                  frame "wait3" {
                    n916 = local read "Time Between Launches"() -> (w1227:dbl)
                    n917 = local read "Launch Wait Time"() -> (w1230:dbl)
                    n918 = local read "Time Between tick"() -> (w1229:dbl)
                    n919 = local read "Charge Up Time"() -> (w1231:dbl)
                    n920 = Multiply(x=3.0, y=w1230) -> (x*y=w1226:dbl)
                    n921 = Multiply(x=2.0, y=w1227) -> (x*y=w1224:dbl)
                    n922 = Compound Arithmetic op=ADD(w1229, w1231, w1226, w1224) -> (w1228:dbl)
                    n923 = Tick Count (ms)() -> (millisecond timer value=w1233:u32)
                    n924 = Less Or Equal?(x=w1228, y=w1233) -> (x <= y?=w1232:bool)
                    n925 = Select(t=T1."Fire 4", s=w1232, f=T1."wait3") -> (s? t:f=w1236:T1)
                    n926 = local write "Quicklaunch State"(w1236) -> ()
                  }
                  frame "Fire 4" {
                    w1238 = 3.0 ("y")
                    n927 = local read "Time Between Launches"() -> (w1241:dbl)
                    n928 = local write "Quicklaunch State"(T1."Fire 4" ("Quicklaunch State")) -> ()
                    n929 = local read "Launch Wait Time"() -> (w1242:dbl)
                    n930 = local read "Launch Wait tick"() -> (w1245:dbl)
                    n931 = local read "Charge Up Time"() -> (w1244:dbl)
                    n932 = Multiply(x=w1242, y=w1238) -> (x*y=w1239:dbl)
                    n933 = Multiply(x=w1241, y=w1238) -> (x*y=w1240:dbl)
                    n934 = Compound Arithmetic op=ADD(w1245, w1244, w1239, w1240) -> (w1243:dbl)
                    n935 = Tick Count (ms)() -> (millisecond timer value=w1252:u32)
                    n936 = Less Or Equal?(x=w1243, y=w1252) -> (x <= y?=w1249:bool)
                    n937 = Select(t=WPI_SolenoidValue."Reverse" ("Value"), s=w1249, f=WPI_SolenoidValue."Forward" ("Value")) -> (s? t:f=w1246:T8)
                    n938 = call <vilib>:"WPI_SolenoidRefNum Registry Get.vi"("refnum name"="Launch Cylinder") -> ("SolenoidDevRef"=w1251:T20)  [unwired: 9 in, 1 out]
                    n939 = call-poly <vilib>:"WPI_SolenoidSet.vi"("Value"=w1246, "SolenoidDevRef"=w1251) -> ()  [unwired: 8 in, 2 out]
                  }
                }
                n940 = local read "Auton Launch Reduction"() -> (w1132:dbl)
                n941 = Subtract(x=1.0, y=w1132) -> (x-y=w1136:dbl)
                n942 = In Range and Coerce(upper limit=1.0, x=w1136, lower limit=0.0 ("x")) -> (coerced(x)=w1133:dbl)  [unwired: 1 out]
                n943 = Divide(x=w1133, y="Fast-Slow Variable") -> (x/y=w1141:dbl)
                n944 = Negate(x=w1133) -> (-x=w1140:dbl)
                n945 = call <vilib>:"WPI_MotorControlRefNum Registry Get.vi"("refnum name"="Launch Motor Fast") -> ("error out"=w1143:errorcluster, "MotorControlDevRef"=w1144:T10)  [unwired: 9 in]
                n946 = call <vilib>:"WPI_MotorControlSetOutput.vi"("error in (no error)"=w1143, "Output"=w1140, "MotorControlDevRef"=w1144) -> ()  [unwired: 6 in, 3 out]
                n947 = Negate(x=w1141) -> (-x=w1139:dbl)
                n948 = call <vilib>:"WPI_MotorControlRefNum Registry Get.vi"("refnum name"="Launch Motor Slow") -> ("error out"=w1146:errorcluster, "MotorControlDevRef"=w1145:T10)  [unwired: 9 in]
                n949 = call <vilib>:"WPI_MotorControlSetOutput.vi"("error in (no error)"=w1146, "Output"=w1139, "MotorControlDevRef"=w1145) -> ()  [unwired: 6 in, 3 out]
              }
            }
          }
        }
        frame "Middle" {
          n950 = flat-sequence {
            frame #0 {
              n951 = while {
                stop <- w1253 stop-if-true
                n952 = stacked-sequence {
                  tunnel: [_ w1265] -> w1253
                  frame #0 {
                    n953 = local read "Numeric 0"() -> (w1261:dbl)
                    n954 = Tick Count (ms)() -> (millisecond timer value=w1262:u32)
                    n955 = First Call?() -> (First Call?: T/F=w1263:bool)
                    n956 = Select(t=w1262, s=w1263, f=w1261) -> (s? t:f=w1260:dbl)
                    n957 = local write "Numeric 0"(w1260) -> ()
                  }
                  frame #1 {
                    n958 = local read "Drive wait time cl"() -> (w1264:dbl)
                    n959 = local read "Numeric 0"() -> (w1268:dbl)
                    n960 = Add(x=w1264, y=w1268) -> (x+y=w1267:dbl)
                    n961 = Tick Count (ms)() -> (millisecond timer value=w1266:u32)
                    n962 = Less?(x=w1267, y=w1266) -> (x < y?=w1265:bool)
                  }
                }
                n963 = call <vilib>:"WPI_RobotDriveRefNum Registry Get.vi"("refnum name"="Left and Right Motors") -> ("RobotDriveDevRef"=w1258:T9)  [unwired: 1 in, 9 out]
                n964 = call <vilib>:"WPI_RobotDriveArcadeDrive_Standard(NoSaturation).vi"("Y axis value"=1.0 ("X axis value"), "X axis value"=0.0, "RobotDriveDevRef"=w1258) -> ("Motor Values"=w1256:dbl[])  [unwired: 1 in, 7 out]
                n965 = call <vilib>:"SD Write Numeric Array.vi"("Numeric Array"=w1256, "Name"="RobotDrive Motors") -> ()  [unwired: 8 in, 2 out]
              }
            }
            frame #1 {
              n966 = local read "Time between launches"() -> (w1272:dbl)
              n967 = local read "Launch Wait Time"() -> (w1273:dbl)
              n968 = local read "Charge Up Time"() -> (w1274:dbl)
              n969 = Tick Count (ms)() -> (millisecond timer value=w1275:u32)
              n970 = Add(x=w1275, y=w1274) -> (x+y=w1269:dbl)
              n971 = Add(x=w1275, y=w1273) -> (x+y=w1270:dbl)
              n972 = Add(x=w1275, y=w1272) -> (x+y=w1271:dbl)
              n973 = local write "Time Between tick"(w1271) -> ()
              n974 = local write "Launch Wait tick"(w1270) -> ()
              n975 = local write "Charge Up tick"(w1269) -> ()
            }
            frame #2 {
              n976 = while {
                stop <- FALSE stop-if-true
                n977 = local read "Quicklaunch State"() -> (w1283:T1)
                n978 = case shown="\"Charge Up \"" w1283 {
                  frame "Charge Up " {
                    n979 = local read "Charge Up tick"() -> (w1294:dbl)
                    n980 = Tick Count (ms)() -> (millisecond timer value=w1298:u32)
                    n981 = Less Or Equal?(x=w1294, y=w1298) -> (x <= y?=w1297:bool)
                    n982 = Select(t=T1."Fire 1", s=w1297, f=T1."Charge Up ") -> (s? t:f=w1299:T1)
                    n983 = local write "Quicklaunch State"(w1299) -> ()
                  }
                  frame "Fire 1" {
                    n984 = local read "Launch Wait tick"() -> (w1308:dbl)
                    n985 = local read "Charge Up Time"() -> (w1306:dbl)
                    n986 = Add(x=w1308, y=w1306) -> (x+y=w1307:dbl)
                    n987 = Tick Count (ms)() -> (millisecond timer value=w1312:u32)
                    n988 = Less Or Equal?(x=w1307, y=w1312) -> (x <= y?=w1303:bool)
                    n989 = Select(t=WPI_SolenoidValue."Reverse" ("Value"), s=w1303, f=WPI_SolenoidValue."Forward" ("Value")) -> (s? t:f=w1300:T8)
                    n990 = call <vilib>:"WPI_SolenoidRefNum Registry Get.vi"("refnum name"="Launch Cylinder") -> ("SolenoidDevRef"=w1305:T20)  [unwired: 9 in, 1 out]
                    n991 = call-poly <vilib>:"WPI_SolenoidSet.vi"("Value"=w1300, "SolenoidDevRef"=w1305) -> ()  [unwired: 8 in, 2 out]
                    n992 = Select(t=T1."wait1", s=w1303, f=T1."Fire 1") -> (s? t:f=w1311:T1)
                    n993 = local write "Quicklaunch State"(w1311) -> ()
                  }
                  frame "wait1" {
                    n994 = local read "Time Between tick"() -> (w1315:dbl)
                    n995 = local read "Launch Wait Time"() -> (w1313:dbl)
                    n996 = local read "Charge Up Time"() -> (w1316:dbl)
                    n997 = Compound Arithmetic op=ADD(w1315, w1316, w1313) -> (w1314:dbl)
                    n998 = Tick Count (ms)() -> (millisecond timer value=w1318:u32)
                    n999 = Less Or Equal?(x=w1314, y=w1318) -> (x <= y?=w1317:bool)
                    n1000 = Select(t=T1."Fire 2", s=w1317, f=T1."wait1") -> (s? t:f=w1321:T1)
                    n1001 = local write "Quicklaunch State"(w1321) -> ()
                  }
                  frame "Fire 2" {
                    n1002 = local read "Time Between Launches"() -> (w1323:dbl)
                    n1003 = local read "Launch Wait Time"() -> (w1324:dbl)
                    n1004 = local read "Launch Wait tick"() -> (w1326:dbl)
                    n1005 = local read "Charge Up Time"() -> (w1325:dbl)
                    n1006 = Compound Arithmetic op=ADD(w1326, w1325, w1324, w1323) -> (w1322:dbl)
                    n1007 = Tick Count (ms)() -> (millisecond timer value=w1336:u32)
                    n1008 = Less Or Equal?(x=w1322, y=w1336) -> (x <= y?=w1330:bool)
                    n1009 = Select(t=WPI_SolenoidValue."Reverse" ("Value"), s=w1330, f=WPI_SolenoidValue."Forward" ("Value")) -> (s? t:f=w1327:T8)
                    n1010 = call <vilib>:"WPI_SolenoidRefNum Registry Get.vi"("refnum name"="Launch Cylinder") -> ("SolenoidDevRef"=w1332:T20)  [unwired: 9 in, 1 out]
                    n1011 = call-poly <vilib>:"WPI_SolenoidSet.vi"("Value"=w1327, "SolenoidDevRef"=w1332) -> ()  [unwired: 8 in, 2 out]
                    n1012 = Select(t=T1."wait2", s=w1330, f=T1."Fire 2") -> (s? t:f=w1335:T1)
                    n1013 = local write "Quicklaunch State"(w1335) -> ()
                  }
                  frame "wait2" {
                    n1014 = local read "Launch Wait Time"() -> (w1342:dbl)
                    n1015 = local read "Time Between Launches"() -> (w1339:dbl)
                    n1016 = local read "Time Between tick"() -> (w1341:dbl)
                    n1017 = local read "Charge Up Time"() -> (w1343:dbl)
                    n1018 = Multiply(x=2.0, y=w1342) -> (x*y=w1338:dbl)
                    n1019 = Compound Arithmetic op=ADD(w1341, w1343, w1338, w1339) -> (w1340:dbl)
                    n1020 = Tick Count (ms)() -> (millisecond timer value=w1345:u32)
                    n1021 = Less Or Equal?(x=w1340, y=w1345) -> (x <= y?=w1344:bool)
                    n1022 = Select(t=T1."Fire 3", s=w1344, f=T1."wait2") -> (s? t:f=w1348:T1)
                    n1023 = local write "Quicklaunch State"(w1348) -> ()
                  }
                  frame "Fire 3" {
                    w1349 = 2.0 ("y")
                    n1024 = local read "Time Between Launches"() -> (w1352:dbl)
                    n1025 = local read "Launch Wait Time"() -> (w1353:dbl)
                    n1026 = local read "Launch Wait tick"() -> (w1356:dbl)
                    n1027 = local read "Charge Up Time"() -> (w1355:dbl)
                    n1028 = Multiply(x=w1353, y=w1349) -> (x*y=w1350:dbl)
                    n1029 = Multiply(x=w1352, y=w1349) -> (x*y=w1351:dbl)
                    n1030 = Compound Arithmetic op=ADD(w1356, w1355, w1350, w1351) -> (w1354:dbl)
                    n1031 = Tick Count (ms)() -> (millisecond timer value=w1366:u32)
                    n1032 = Less Or Equal?(x=w1354, y=w1366) -> (x <= y?=w1360:bool)
                    n1033 = Select(t=WPI_SolenoidValue."Reverse" ("Value"), s=w1360, f=WPI_SolenoidValue."Forward" ("Value")) -> (s? t:f=w1357:T8)
                    n1034 = call <vilib>:"WPI_SolenoidRefNum Registry Get.vi"("refnum name"="Launch Cylinder") -> ("SolenoidDevRef"=w1362:T20)  [unwired: 9 in, 1 out]
                    n1035 = call-poly <vilib>:"WPI_SolenoidSet.vi"("Value"=w1357, "SolenoidDevRef"=w1362) -> ()  [unwired: 8 in, 2 out]
                    n1036 = Select(t=T1."wait3", s=w1360, f=T1."Fire 3") -> (s? t:f=w1365:T1)
                    n1037 = local write "Quicklaunch State"(w1365) -> ()
                  }
                  frame "wait3" {
                    n1038 = local read "Time Between Launches"() -> (w1371:dbl)
                    n1039 = local read "Launch Wait Time"() -> (w1374:dbl)
                    n1040 = local read "Time Between tick"() -> (w1373:dbl)
                    n1041 = local read "Charge Up Time"() -> (w1375:dbl)
                    n1042 = Multiply(x=3.0, y=w1374) -> (x*y=w1370:dbl)
                    n1043 = Multiply(x=2.0, y=w1371) -> (x*y=w1368:dbl)
                    n1044 = Compound Arithmetic op=ADD(w1373, w1375, w1370, w1368) -> (w1372:dbl)
                    n1045 = Tick Count (ms)() -> (millisecond timer value=w1377:u32)
                    n1046 = Less Or Equal?(x=w1372, y=w1377) -> (x <= y?=w1376:bool)
                    n1047 = Select(t=T1."Fire 4", s=w1376, f=T1."wait3") -> (s? t:f=w1380:T1)
                    n1048 = local write "Quicklaunch State"(w1380) -> ()
                  }
                  frame "Fire 4" {
                    w1382 = 3.0 ("y")
                    n1049 = local read "Time Between Launches"() -> (w1385:dbl)
                    n1050 = local write "Quicklaunch State"(T1."Fire 4" ("Quicklaunch State")) -> ()
                    n1051 = local read "Launch Wait Time"() -> (w1386:dbl)
                    n1052 = local read "Launch Wait tick"() -> (w1389:dbl)
                    n1053 = local read "Charge Up tick"() -> (w1388:dbl)
                    n1054 = Multiply(x=w1386, y=w1382) -> (x*y=w1383:dbl)
                    n1055 = Multiply(x=w1385, y=w1382) -> (x*y=w1384:dbl)
                    n1056 = Compound Arithmetic op=ADD(w1389, w1388, w1383, w1384) -> (w1387:dbl)
                    n1057 = Tick Count (ms)() -> (millisecond timer value=w1396:u32)
                    n1058 = Less Or Equal?(x=w1387, y=w1396) -> (x <= y?=w1393:bool)
                    n1059 = Select(t=WPI_SolenoidValue."Reverse" ("Value"), s=w1393, f=WPI_SolenoidValue."Forward" ("Value")) -> (s? t:f=w1390:T8)
                    n1060 = call <vilib>:"WPI_SolenoidRefNum Registry Get.vi"("refnum name"="Launch Cylinder") -> ("SolenoidDevRef"=w1395:T20)  [unwired: 9 in, 1 out]
                    n1061 = call-poly <vilib>:"WPI_SolenoidSet.vi"("Value"=w1390, "SolenoidDevRef"=w1395) -> ()  [unwired: 8 in, 2 out]
                  }
                }
                n1062 = Subtract(x=1.0, y="Auton Launch Reduction") -> (x-y=w1280:dbl)
                n1063 = In Range and Coerce(upper limit=1.0, x=w1280, lower limit=0.0 ("x")) -> (coerced(x)=w1276:dbl)  [unwired: 1 out]
                n1064 = local read "Fast-Slow Variable"() -> (w1282:dbl)
                n1065 = Divide(x=w1276, y=w1282) -> (x/y=w1287:dbl)
                n1066 = Negate(x=w1276) -> (-x=w1286:dbl)
                n1067 = call <vilib>:"WPI_MotorControlRefNum Registry Get.vi"("refnum name"="Launch Motor Fast") -> ("error out"=w1289:errorcluster, "MotorControlDevRef"=w1290:T10)  [unwired: 9 in]
                n1068 = call <vilib>:"WPI_MotorControlSetOutput.vi"("error in (no error)"=w1289, "Output"=w1286, "MotorControlDevRef"=w1290) -> ()  [unwired: 6 in, 3 out]
                n1069 = Negate(x=w1287) -> (-x=w1285:dbl)
                n1070 = call <vilib>:"WPI_MotorControlRefNum Registry Get.vi"("refnum name"="Launch Motor Slow") -> ("error out"=w1292:errorcluster, "MotorControlDevRef"=w1291:T10)  [unwired: 9 in]
                n1071 = call <vilib>:"WPI_MotorControlSetOutput.vi"("error in (no error)"=w1292, "Output"=w1285, "MotorControlDevRef"=w1291) -> ()  [unwired: 6 in, 3 out]
              }
            }
          }
        }
      }
    }
  }
  n1072 = while {
    stop <- FALSE stop-if-true
    n1073 = call <vilib>:"WPI_RelayRefNum Registry Get.vi"("refnum name"="Compresser") -> ("error out"=w1401:errorcluster, "RelayDevRef"=w1400:T24)  [unwired: 9 in]
    n1074 = call <vilib>:"WPI_RelaySet.vi"("error in (no error)"=w1401, "RelayValue"=WPI_RelayValue."Forward", "RelayDevRef"=w1400) -> ()  [unwired: 7 in, 2 out]
  }
  n1075 = disable-structure shown="Disabled" {
    frame Disabled {
      # "This sample code describes robot movements in an array. You can extend it to control other motors\non your robot. You can also use file I/O to move the data to a text file."
      n1076 = call <vilib>:"WPI_RobotDriveRefNum Registry Get.vi"("refnum name"="Left and Right Motors") -> ("RobotDriveDevRef"=w1403:T9)  [unwired: 1 in, 9 out]
      n1077 = for {
        shift-right: [w1409] -> _
        shift-left: w1403 -> [w1410]
        tunnel: "Array of robot movements" -> [w1405] mode=indexing
        n1078 = Unbundle By Name(w1405) -> ("X Joystick Value"=w1408:dbl, "Y Joystick Value"=w1407:dbl, "Delay (sec)"=w1406:dbl)  [unwired: 1 out]
        n1079 = call-poly <vilib>:"WPI_RobotDriveArcadeDrive.vi"("Y axis value"=w1407, "X axis value"=w1408, "RobotDriveDevRef"=w1410) -> ("Motor Values"=w1412:dbl[], "RobotDriveDevRef"=w1411:T9)  [unwired: 1 in, 6 out]
        n1080 = call <vilib>:"SD Write Numeric Array.vi"("Numeric Array"=w1412, "Name"="RobotDrive Motors") -> ()  [unwired: 8 in, 2 out]
        n1081 = call <vilib>:"WPI_RobotDriveDelayAndUpdateSafety.vi"("Delay (s)"=w1406, "RobotDriveDevRef"=w1411) -> ("RobotDriveDevRef 2"=w1409:T9)  [unwired: 8 in, 1 out]
        "Current Movement, for debugging" <- w1405
      }
    }
    frame Enabled {
    }
  }
  n1082 = disable-structure shown="Enabled" {
    frame Disabled {
      w1414 = "RobotDrive Motors" ("Name")
      # "This is some simple sample code to drive your robot curving one direction and then the other."
      # "stand still"
      # "turn left for 0.5 second"
      # "turn right for 1 second"
      n1083 = call <vilib>:"WPI_RobotDriveRefNum Registry Get.vi"("refnum name"="Left and Right Motors") -> ("RobotDriveDevRef"=w1418:T9)  [unwired: 1 in, 9 out]
      n1084 = call-poly <vilib>:"WPI_RobotDriveArcadeDrive.vi"("Y axis value"=0.5 ("X axis value"), "X axis value"=0.25, "RobotDriveDevRef"=w1418) -> ("Motor Values"=w1417:dbl[], "RobotDriveDevRef"=w1425:T9)  [unwired: 1 in, 6 out]
      n1085 = call <vilib>:"SD Write Numeric Array.vi"("Numeric Array"=w1417, "Name"=w1414) -> ()  [unwired: 8 in, 2 out]
      n1086 = call <vilib>:"WPI_RobotDriveDelayAndUpdateSafety.vi"("Delay (s)"=1.0, "RobotDriveDevRef"=w1425) -> ("RobotDriveDevRef 2"=w1424:T9)  [unwired: 8 in, 1 out]
      n1087 = call-poly <vilib>:"WPI_RobotDriveArcadeDrive.vi"("Y axis value"=0.25 ("X axis value"), "X axis value"=0.5, "RobotDriveDevRef"=w1424) -> ("Motor Values"=w1416:dbl[], "RobotDriveDevRef"=w1423:T9)  [unwired: 1 in, 6 out]
      n1088 = call <vilib>:"SD Write Numeric Array.vi"("Numeric Array"=w1416, "Name"=w1414) -> ()  [unwired: 8 in, 2 out]
      n1089 = call <vilib>:"WPI_RobotDriveDelayAndUpdateSafety.vi"("Delay (s)"=0.5, "RobotDriveDevRef"=w1423) -> ("RobotDriveDevRef 2"=w1422:T9)  [unwired: 8 in, 1 out]
      n1090 = call-poly <vilib>:"WPI_RobotDriveArcadeDrive.vi"("Y axis value"=0.0 ("X axis value"), "X axis value"=0.0, "RobotDriveDevRef"=w1422) -> ("Motor Values"=w1415:dbl[])  [unwired: 1 in, 7 out]
      n1091 = call <vilib>:"SD Write Numeric Array.vi"("Numeric Array"=w1415, "Name"=w1414) -> ()  [unwired: 8 in, 2 out]
    }
    frame Enabled {
    }
  }
